vi "AutoFocus Loop.vi"(8 "error in":errorcluster, 9 "IBM OptoElectroMechanics Configuration":T1={"Parameter Analizer"={"Parameter Analyzer VISA Session"="COM1", "Sweeping Time Parameters"={"Integration Time"=0, "Short Integration Time (s)"=1.0, "Long Integration Time (s)"=0.0, "Wait Time Parameter"=1.0}, "Acquisition Mode"=enum."Sweeping Mode", "Status Polling Time (ms)"=0, "Comment"="Test VI", "SMU 1 - Sweeping"={"Start / Offset"=0.0, "Stop / Ratio"=1.0, "Step \n(linear only)"=0.01, "Compliance"=0.1, "Power \nCompliance"=0.0, "Mode"=0, "Function"=0, "Sweep Mode"=FALSE}, "SMU 2 - Sweeping"={"Start / Offset"=0.0, "Stop / Ratio"=1.0, "Step \n(linear only)"=0.01, "Compliance"=0.1, "Power \nCompliance"=0.0, "Mode"=0, "Function"=0, "Sweep Mode"=FALSE}, "SMU 3 - Sweeping"={"Start / Offset"=0.0, "Stop / Ratio"=1.0, "Step \n(linear only)"=0.01, "Compliance"=0.1, "Power \nCompliance"=0.0, "Mode"=0, "Function"=0, "Sweep Mode"=FALSE}, "SMU 4 - Sweeping"={"Start / Offset"=0.0, "Stop / Ratio"=1.0, "Step \n(linear only)"=0.01, "Compliance"=0.1, "Power \nCompliance"=0.0, "Mode"=0, "Function"=0, "Sweep Mode"=FALSE}, "Sweep Spacing"=0, "Range"=0, "SMU1 - Sampling"={"Source"=10.0, "Compliance"=1e-05, "Mode"=0, "Function"=FALSE}, "SMU2 - Sampling"={"Source"=1.0, "Compliance"=1.0, "Mode"=0, "Function"=FALSE}, "SMU3 - Sampling"={"Source"=10.0, "Compliance"=1e-05, "Mode"=0, "Function"=FALSE}, "SMU4 - Sampling"={"Source"=0.1, "Compliance"=60.0, "Mode"=10, "Function"=FALSE}, "Sampling Time Parameters"={"Initial Interval (s)"=0.1, "Number of Samples"=60, "Total Sampling Time (s)"=10.0, "Hold Time (s)"=0.0, "Sampling Mode"=0, "Sampling Time"=0}, "Stop Condition"={"Enable Delay (s)"=0.0, "Name"="", "Threshold"=0.0, "num. of events"=1, "Event"=0, "Stop Condition Enable"=FALSE}}, "Switching Matrix"={"Switching Matrix VISA Session"="GPIB0::18::INSTR", "Connections"=[{"Connections"=[FALSE, FALSE, FALSE, FALSE, FALSE, FALSE, FALSE, FALSE, FALSE, FALSE, FALSE, FALSE], "Connection Type"=enum."Disconnected"}, {"Connections"=[FALSE, FALSE, FALSE, FALSE, FALSE, FALSE, FALSE, FALSE, FALSE, FALSE, FALSE, FALSE], "Connection Type"=enum."Disconnected"}, {"Connections"=[FALSE, FALSE, FALSE, FALSE, FALSE, FALSE, FALSE, FALSE, FALSE, FALSE, FALSE, FALSE], "Connection Type"=enum."Disconnected"}, {"Connections"=[FALSE, FALSE, FALSE, FALSE, FALSE, FALSE, FALSE, FALSE, FALSE, FALSE, FALSE, FALSE], "Connection Type"=enum."Disconnected"}, {"Connections"=[FALSE, FALSE, FALSE, FALSE, FALSE, FALSE, FALSE, FALSE, FALSE, FALSE, FALSE, FALSE], "Connection Type"=enum."Disconnected"}, {"Connections"=[FALSE, FALSE, FALSE, FALSE, FALSE, FALSE, FALSE, FALSE, FALSE, FALSE, FALSE, FALSE], "Connection Type"=enum."Disconnected"}, {"Connections"=[FALSE, FALSE, FALSE, FALSE, FALSE, FALSE, FALSE, FALSE, FALSE, FALSE, FALSE, FALSE], "Connection Type"=enum."Disconnected"}, {"Connections"=[FALSE, FALSE, FALSE, FALSE, FALSE, FALSE, FALSE, FALSE, FALSE, FALSE, FALSE, FALSE], "Connection Type"=enum."Disconnected"}]}, "Stress Control"={"Stress Control VISA Session"="StrainMotor", "Axis"=0, "Motion"=0, "Destination (°)"=0.0, "Speed (°/s)"=4.0, "Position (°)"=25.0}, "Optical Spectrometer"={"Laser Settings"={"Laser Wavelength"=enum."365 nm", "Neutral Density Filter"=enum."100%"}, "Spectrometer Settings"={"Confocal Hole Size (µm)"=0.0, "Grating"=2, "Detector"=enum."InGaAs Array"}, "Acquisition Settings"={"Acquisition Mode"=enum."Multi-Window", "Spectal Position (nm)"=632.0, "From (nm)"=735.0, "To (nm)"=0.0, "Integration Time (s)"=0.0, "Number of Accumulations"=3, "AutoScanning"=FALSE, "Spike Removal"=FALSE}, "Path"=path "C:/07 - Prizes and Awards/Marie Curie Prize/Reply Editors Final NCOMMS(10).docx"}, "Switches & Mirrors"={"Relay VISA Session"="COM1", "Switches"={"Laser"=FALSE, "Video"=FALSE}, "Delays (ms)"={"Laser"=500, "Video"=1500}}, "Camera"={"Settings"={"Pixel clock"=20, "Frame rate"=30.0, "Exposure time"=33.21525, "Master Gain"=0, "Red Gain"=0, "Green Gain"=0, "Blue Gain"=0, "Auto Gain"=FALSE, "White-balance"=FALSE, "Color Correction"=FALSE}}, "XYZ Stage"={"Connection Settings"={"Tango VISA"="", "Baudrate"=57600, "Show Protocol?"=FALSE}, "Manual Control"={"North"=FALSE, "South"=FALSE, "West"=FALSE, "East"=FALSE, "Up"=FALSE, "Down"=FALSE, "Stop"=FALSE, "XY Step"=0.0, "Z step"=0.0}, "Coordinate Control"={"Motion Mode"=enum."Absolute", "Destination [mm]"=[]}}, "AutoFocus"={"Matching Criteria"={"Minimum Score"=700.0, "Color Score Weight"=700.0, "Minimum Contrast"=50, "Match Mode"=0, "Match Feature Mode"=0, "Subpixel Accuracy"=TRUE, "Color Sensitivity"=1, "Search Strategy"=1}, "Z Scan Parameters"={"Z Range"=1380.0, "Resolution"=5000.0, "Initial Direction"=enum."Up", "Focus Threshold"=0.1, "Ascent Constant"=0.1}, "Displacement"=0.0, "Transformation Matrix"=[]}, "Sava Data"={"Workspace Info"={"Device Name"="ProberHead_Tst_C29K3_7(2)", "Device Info"="ProberHead_Tst_C29", "Path"=path "C:/Users/gio/Desktop/ProbeHeadTest"}, "Instrument Configuration"={"Instrument"=enum."Unknown Instrument", "Configuration"="Test Configuration"}, "Stress Motor Position"=0.0, "Electrical Measurement"={"Sequence"=[], "V1"=[], "V2"=[], "V3"=[], "V4"=[], "I1"=[], "I2"=[], "I3"=[], "I4"=[]}, "Optical Spectrum"={"Intensity"=[], "Wavelength"=[], "Energy"=[], "Raman Shift"=[], "Detector Temperature"=0.0}}, "PlotData"={"Sliders"={"Strain Sequence"=0, "Instrument Sequence"=0}, "Measurement"={"Which Instrument?"=enum."No Plot", "Electrical Measurement"={"Sequence"=[], "V1"=[], "V2"=[], "V3"=[], "V4"=[], "I1"=[], "I2"=[], "I3"=[], "I4"=[]}, "Measurement Mode"=enum."Sweeping Mode", "Optical Spectrum"={"Intensity"=[], "Wavelength"=[], "Energy"=[], "Raman Shift"=[], "Detector Temperature"=0.0}}, "Instrument Steps"=[], "Strain Points"=[]}, "Instrument Sequence"={"Caller VI"=enum."User"}, "Strain Measurement"={"Stress Sequence "={"Max Motor Position"=1380.0, "# Intermediate Points"=5000, "Initial Direction"=enum."Tension"}, "Track?"=FALSE}} {"AutoFocus"."Displacement" scale=1.0..1000.0; "AutoFocus"."Z Scan Parameters"."Focus Threshold" min=0.0 max=1000.0 step=1.0 format="%#_2f"; "AutoFocus"."Z Scan Parameters"."Ascent Constant" min=0.0 max=1000.0 step=1.0 format="%#_2f"; "AutoFocus"."Z Scan Parameters"."Resolution" min=0.0 max=1.0 step=0.01 format="%_2g"; "AutoFocus"."Z Scan Parameters"."Z Range" format="%_3g"; "AutoFocus"."Matching Criteria"."Match Mode" items=["Shift Invariant", "Rotation Invariant"]; "AutoFocus"."Matching Criteria"."Match Feature Mode" items=["Color and Shape", "Color", "Shape"]; "AutoFocus"."Matching Criteria"."Color Sensitivity" items=["Low Sensitivity", "Medium Sensitivity", "High Sensitivity"]; "AutoFocus"."Matching Criteria"."Search Strategy" items=["Conservative", "Balance", "Aggressive", "Very Aggressive"]; "XYZ Stage"."Manual Control"."Z step" scale=0.1..10.0; "XYZ Stage"."Manual Control"."XY Step" scale=0.1..1000.0; "Camera"."Settings"."Blue Gain" min=0 max=100 scale=0.0..100.0; "Camera"."Settings"."Green Gain" min=0 max=100 scale=0.0..100.0; "Camera"."Settings"."Red Gain" min=0 max=100 scale=0.0..100.0; "Camera"."Settings"."Master Gain" min=0 max=100 scale=0.0..100.0; "Camera"."Settings"."Exposure time" min=0.101625 max=159.246375 step=0.101625 scale=0.101625..159.246375 scale format="%#.3g"; "Camera"."Settings"."Frame rate" min=2.7455631699174137 max=6.2675785993528725 step=0.000101625 scale=2.7455631699174137..6.2675785993528725 scale format="%^#_3g"; "Camera"."Settings"."Pixel clock" min=5 max=43 scale=5.0..43.0; "PlotData"."Sliders"."Instrument Sequence" scale=0.0..10.0; "PlotData"."Sliders"."Strain Sequence" scale=0.0..10.0; "Strain Measurement"."Stress Sequence"."# Intermediate Points" max=1390; "Parameter Analizer"."Stop Condition"."Event" items=["Value > Threshold", "Value < Threshold", "| Value | > | Threshold |", "| Value | < | Threshold |"]; "Parameter Analizer"."Stop Condition"."Threshold" format="%^.2e"; "Parameter Analizer"."Stop Condition"."Enable Delay (s)" format="%.1f"; "Parameter Analizer"."Sampling Time Parameters"."Sampling Time" items=["Auto (linear only)", "No Limit", "Set Limit"]; "Parameter Analizer"."Sampling Time Parameters"."Sampling Mode" items=["Linear", "Log10", "Log25", "Log50", "Thinned Out"]; "Parameter Analizer"."Sampling Time Parameters"."Hold Time (s)" format="%.4f"; "Parameter Analizer"."Sampling Time Parameters"."Total Sampling Time (s)" format="%.1f"; "Parameter Analizer"."Sampling Time Parameters"."Initial Interval (s)" format="%^.3e"; "Parameter Analizer"."SMU 4 - Sweeping"."Function" items=["Disabled", "Var 1", "Var 2", "Var 1'", "Constant"]; "Parameter Analizer"."SMU 4 - Sweeping"."Mode" items=["V", "I", "V pulse", "I  pulse", "Common"]; "Parameter Analizer"."SMU 4 - Sweeping"."Power \nCompliance" format="%^.2e"; "Parameter Analizer"."SMU 4 - Sweeping"."Compliance" format="%^.2e"; "Parameter Analizer"."SMU 4 - Sweeping"."Step \n(linear only)" format="%^.4e"; "Parameter Analizer"."SMU 4 - Sweeping"."Stop / Ratio" format="%^.4e"; "Parameter Analizer"."SMU 4 - Sweeping"."Start / Offset" format="%^.4e"; "Parameter Analizer"."SMU 3 - Sweeping"."Function" items=["Disabled", "Var 1", "Var 2", "Var 1'", "Constant"]; "Parameter Analizer"."SMU 3 - Sweeping"."Mode" items=["V", "I", "V pulse", "I  pulse", "Common"]; "Parameter Analizer"."SMU 3 - Sweeping"."Power \nCompliance" format="%^.2e"; "Parameter Analizer"."SMU 3 - Sweeping"."Compliance" format="%^.2e"; "Parameter Analizer"."SMU 3 - Sweeping"."Step \n(linear only)" format="%^.4e"; "Parameter Analizer"."SMU 3 - Sweeping"."Stop / Ratio" format="%^.4e"; "Parameter Analizer"."SMU 3 - Sweeping"."Start / Offset" format="%^.4e"; "Parameter Analizer"."SMU 2 - Sweeping"."Function" items=["Disabled", "Var 1", "Var 2", "Var 1'", "Constant"]; "Parameter Analizer"."SMU 2 - Sweeping"."Mode" items=["V", "I", "V pulse", "I  pulse", "Common"]; "Parameter Analizer"."SMU 2 - Sweeping"."Power \nCompliance" format="%^.2e"; "Parameter Analizer"."SMU 2 - Sweeping"."Compliance" format="%^.2e"; "Parameter Analizer"."SMU 2 - Sweeping"."Step \n(linear only)" format="%^.4e"; "Parameter Analizer"."SMU 2 - Sweeping"."Stop / Ratio" format="%^.4e"; "Parameter Analizer"."SMU 2 - Sweeping"."Start / Offset" format="%^.4e"; "Parameter Analizer"."SMU 1 - Sweeping"."Function" items=["Disabled", "Var 1", "Var 2", "Var 1'", "Constant"]; "Parameter Analizer"."SMU 1 - Sweeping"."Mode" items=["V", "I", "V pulse", "I  pulse", "Common"]; "Parameter Analizer"."SMU 1 - Sweeping"."Power \nCompliance" format="%^.2e"; "Parameter Analizer"."SMU 1 - Sweeping"."Compliance" format="%^.2e"; "Parameter Analizer"."SMU 1 - Sweeping"."Step \n(linear only)" format="%^.4e"; "Parameter Analizer"."SMU 1 - Sweeping"."Stop / Ratio" format="%^.4e"; "Parameter Analizer"."SMU 1 - Sweeping"."Start / Offset" format="%^.4e"; "Parameter Analizer"."Sweeping Time Parameters"."Long Integration Time (s)" scale=0.02..2.0; "Parameter Analizer"."Sweeping Time Parameters"."Short Integration Time (s)" scale=8e-05..0.00192; "Parameter Analizer"."Sweeping Time Parameters"."Integration Time" items=["Short", "Long"]; "Parameter Analizer"."Sweeping Time Parameters"."Wait Time Parameter" format="%.1f"; "Parameter Analizer"."SMU4 - Sampling"."Mode" items=["V", "I", "Common"]; "Parameter Analizer"."SMU4 - Sampling"."Compliance" format="%^.2e"; "Parameter Analizer"."SMU4 - Sampling"."Source" format="%^.3e"; "Parameter Analizer"."SMU3 - Sampling"."Mode" items=["V", "I", "Common"]; "Parameter Analizer"."SMU3 - Sampling"."Compliance" format="%^.2e"; "Parameter Analizer"."SMU3 - Sampling"."Source" format="%^.3e"; "Parameter Analizer"."SMU2 - Sampling"."Mode" items=["V", "I", "Common"]; "Parameter Analizer"."SMU2 - Sampling"."Compliance" format="%^.2e"; "Parameter Analizer"."SMU2 - Sampling"."Source" format="%^.3e"; "Parameter Analizer"."SMU1 - Sampling"."Mode" items=["V", "I", "Common"]; "Parameter Analizer"."SMU1 - Sampling"."Compliance" format="%^.2e"; "Parameter Analizer"."SMU1 - Sampling"."Source" format="%^.3e"; "Parameter Analizer"."Range" items=["auto", "fixed", "limited"]; "Parameter Analizer"."Sweep Spacing" items=["linear", "log 10", "log 25", "log 50"]; "Stress Control"."Axis" min=1 max=3; "Stress Control"."Position (°)" format="%.6g"; "Stress Control"."Speed (°/s)" min=0.0 max=4.0 format="%.6f"; "Stress Control"."Destination (°)" min=-2000000000.0 max=2000000000.0 format="%.6f"; "Stress Control"."Motion" items=["Absolute", "Relative"]; "Optical Spectrometer"."Spectrometer Settings"."Grating" items=["1800 l/mm", "150 l/mm"]}, 10 "Message Queues out":T57, 11 "Notifiers":T44) -> (0 "error out":errorcluster)   [LabVIEW 2014]
uses:
  support/Message Queue/All Message Queues.ctl
  support/Message Queue/Message Cluster.ctl
  support/Notifiers/Notifiers.ctl
  support/Message Handler Loop Notifiers.ctl
  Hardware Control/Parameter Analyzer/Parameter Analyzer Notifiers.ctl
  Hardware Control/Switching Matrix/Switching Matrix Notifiers.ctl
  Hardware Control/Stress Control/StressControl Notifiers.ctl
  Hardware Control/Spectrometer/Spectrometer Notifiers.ctl
  Hardware Control/Switches and Mirrors/SwitchesMirrors Notifiers.ctl
  Hardware Control/Camera/Camera Notifiers.ctl
  Hardware Control/XYZ Stage/XYZ Notifications.ctl
  Hardware Control/Autofocus/Autofocus Notifiers.ctl
  Measurements/Optoelectronic Measurement/Optoelectronic Notifiers.ctl
  Measurements/Save Data/SaveData Notifiers.ctl
  Measurements/Instrument Sequence/Instrument Sequence Notifiers.ctl
  support/Configuration/Configuration.ctl
  Hardware Control/Parameter Analyzer/Parameter Analyzer Config.ctl
  Hardware Control/Parameter Analyzer/Parameter Analyzer Integration Parameters.ctl
  Hardware Control/Parameter Analyzer/Parameter Analyzer SMU Sweeping.ctl
  Hardware Control/Parameter Analyzer/Parameter Analyzer Sweep Spacing.ctl
  Hardware Control/Parameter Analyzer/Parameter Analyzer SMU Range.ctl
  Hardware Control/Parameter Analyzer/Parameter Analyzer SMU Sampling.ctl
  Hardware Control/Parameter Analyzer/Parameter Analyzer Sampling Parameters.ctl
  Hardware Control/Parameter Analyzer/Parameter Analyzer Stop Sampling Conditions.ctl
  Hardware Control/Switching Matrix/Switching Matrix Config.ctl
  Hardware Control/Stress Control/StressControl Config.ctl
  Hardware Control/Spectrometer/Spectrometer Config.ctl
  Hardware Control/Spectrometer/Laser Settings.ctl
  Hardware Control/Spectrometer/Laser.ctl
  Hardware Control/Spectrometer/Filter.ctl
  Hardware Control/Spectrometer/Grating Detector Settings.ctl
  Hardware Control/Spectrometer/Grating.ctl
  Hardware Control/Spectrometer/Detector.ctl
  Hardware Control/Spectrometer/Acquisition Settings.ctl
  Hardware Control/Switches and Mirrors/SwitchesMirrors Config.ctl
  Hardware Control/Switches and Mirrors/SwitchesMirrors Status.ctl
  Hardware Control/Camera/Camera Config.ctl
  Hardware Control/Camera/Camera Settings.ctl
  Hardware Control/XYZ Stage/XYZ Config.ctl
  Hardware Control/XYZ Stage/XYZ Connection Settings.ctl
  Hardware Control/XYZ Stage/XYZ Stage Control.ctl
  Hardware Control/XYZ Stage/XYZ Coordinate Control.ctl
  Hardware Control/Autofocus/AutoFocus Config.ctl
  Hardware Control/Autofocus/ZScan.ctl
  <vilib>/Analysis/Matrix/Datatypes/RealMatrix.ctl
  Measurements/Save Data/SaveData Config.ctl
  Measurements/Save Data/SaveData Workspace Info.ctl
  Measurements/Save Data/SaveData Instrument Configuration.ctl
  Measurements/Instrument Sequence/Instrument List.ctl
  Hardware Control/Spectrometer/Spectral Data.ctl
  Measurements/Plot Data/PlotData Config.ctl
  Measurements/Plot Data/Measurement.ctl
  Measurements/Plot Data/WhichInstrument.ctl
  Hardware Control/Parameter Analyzer/Electrical Data.ctl
  Measurements/Instrument Sequence/Instrument Steps.ctl
  Measurements/Instrument Sequence/Action.ctl
  Measurements/Instrument Sequence/Instrument Sequence Config.ctl
  Measurements/Strain Measurement/Strain Measurement Config.ctl
  Hardware Control/Autofocus/AutoFocus Functions.ctl
  support/Message Queue/Message Queue.lvlib
  <vilib>/Analysis/Matrix/NI_Matrix.lvlib
panel:
  # "LICENSED MATERIALS – PROPERTY OF IBM\nCopyright IBM Corp. 2016,\nALL RIGHTS RESERVED"
  # "XY"
  # "Z"
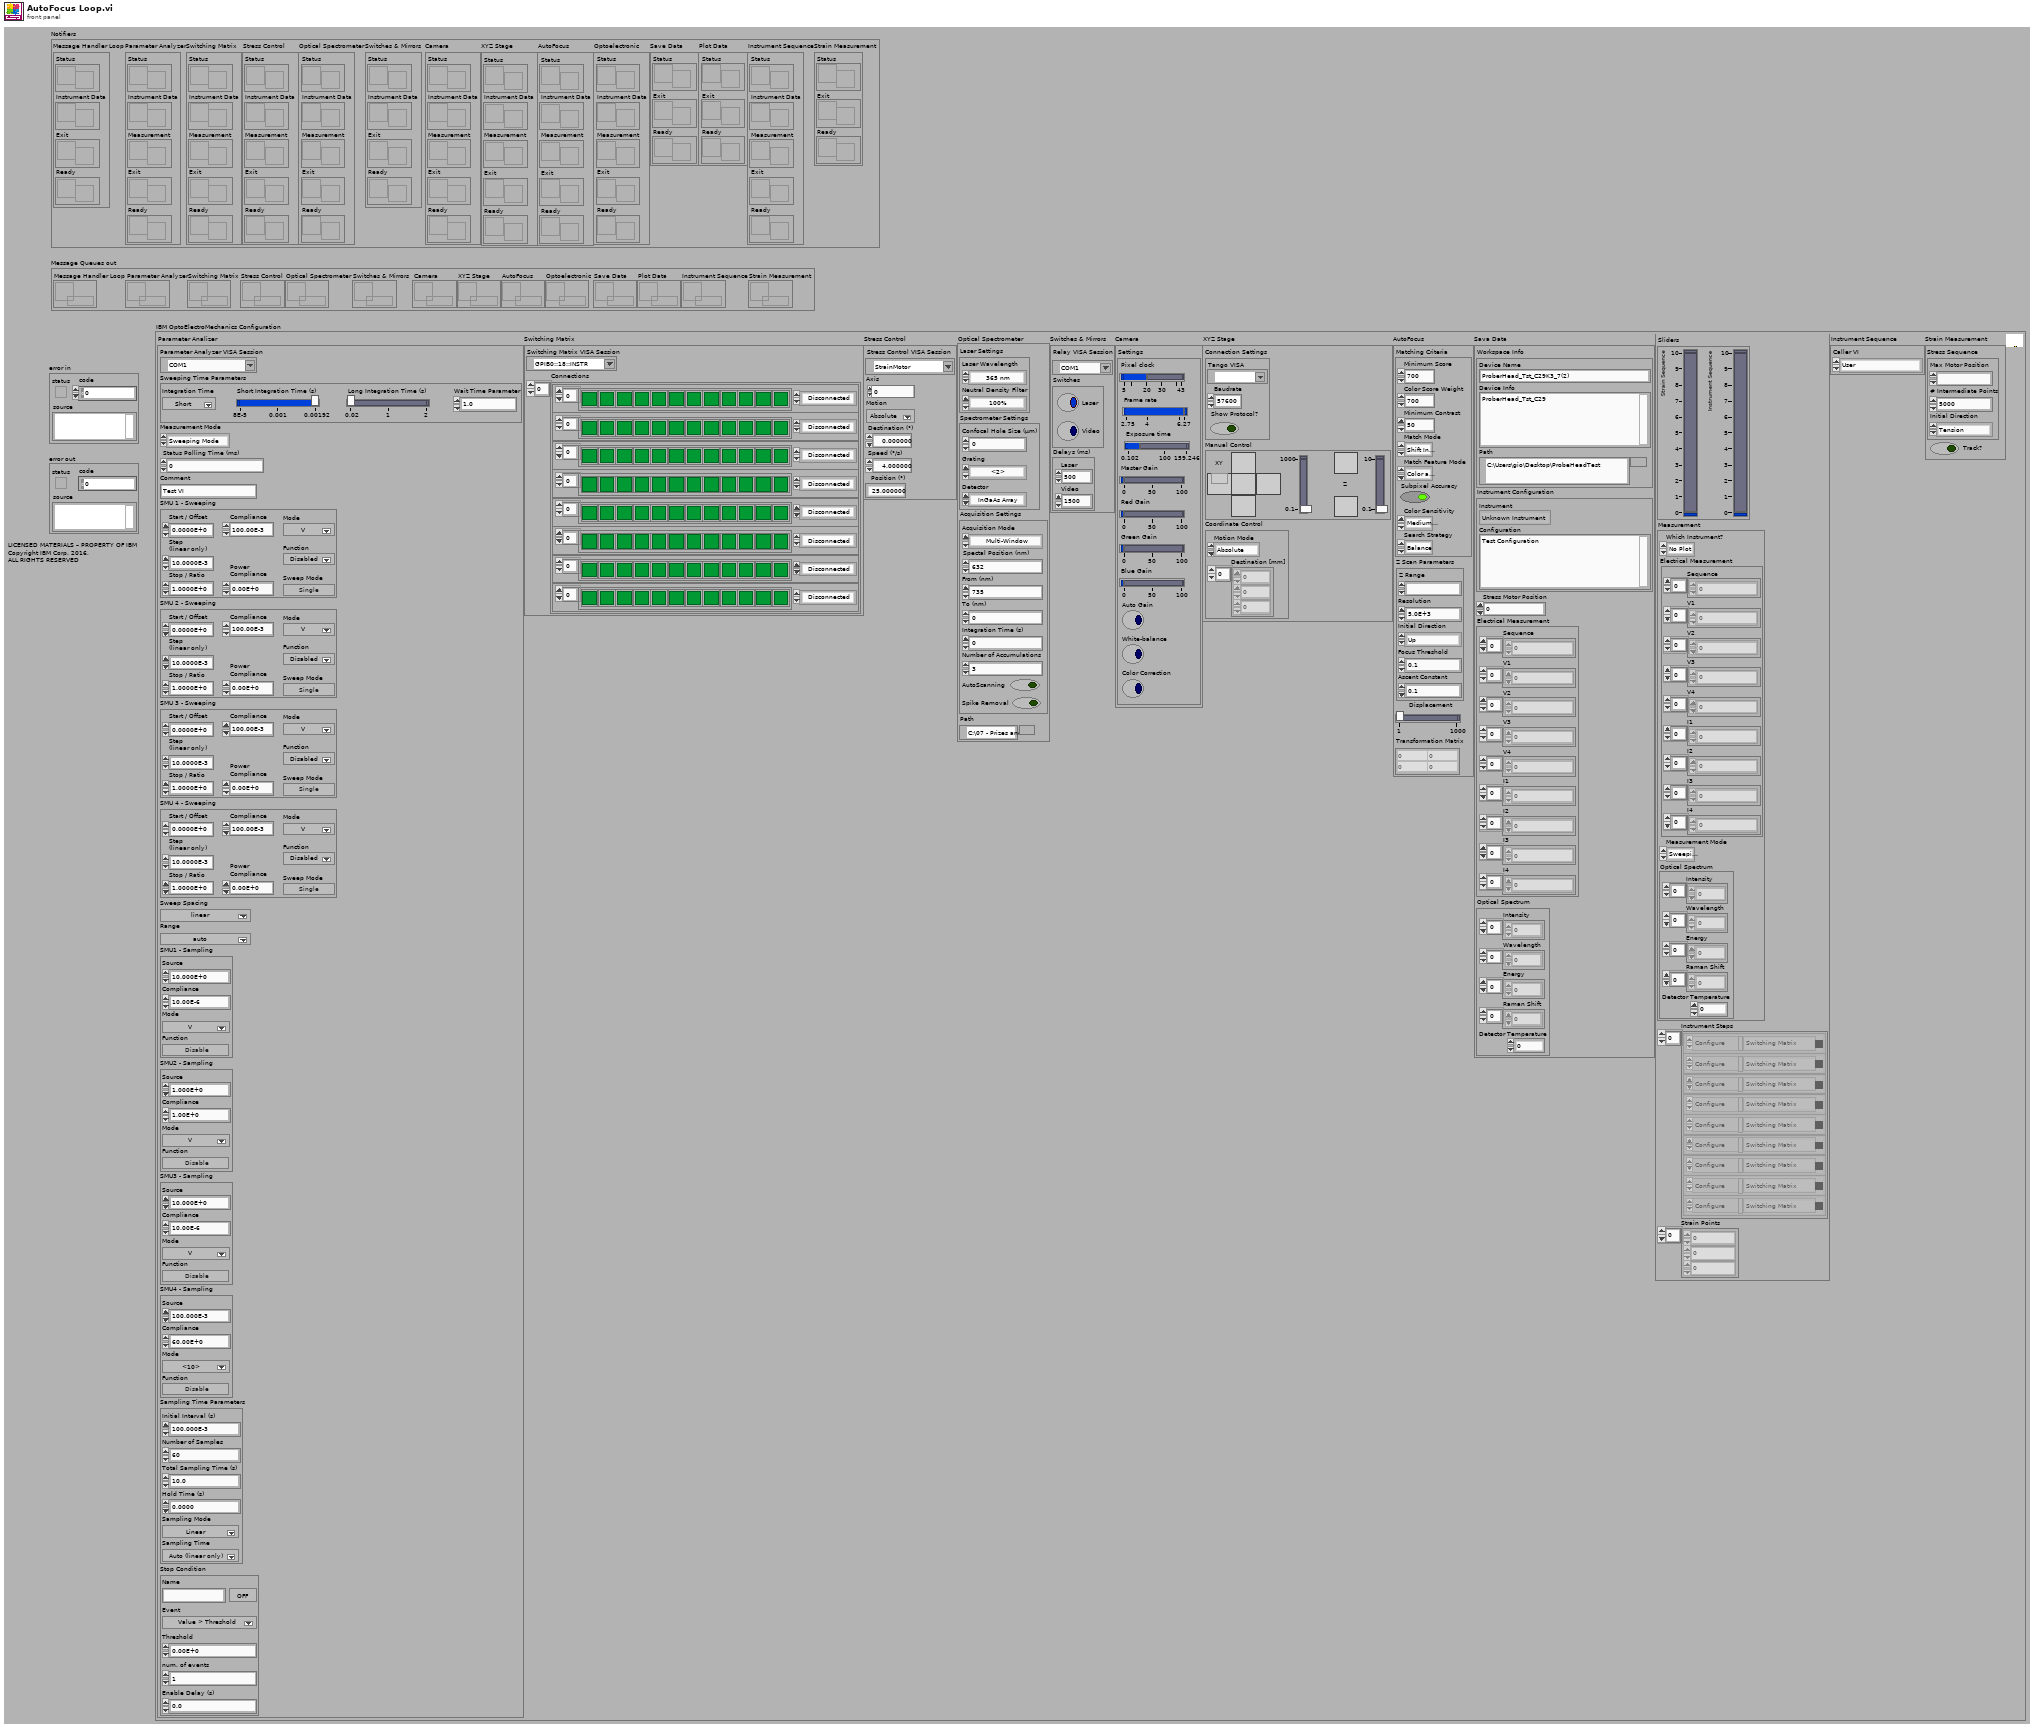
[diagram p1: front panel]
types:
  T1 = typedef "Configuration.ctl" = cluster{"Parameter Analizer":T2, "Switching Matrix":T10, "Stress Control":T11, "Optical Spectrometer":T12, "Switches & Mirrors":T20, "Camera":T22, "XYZ Stage":T24, "AutoFocus":T28, "Sava Data":T31, "PlotData":T36, "Instrument Sequence":T42, "Strain Measurement":T43}
  T2 = typedef "Parameter Analyzer Config.ctl" = cluster{"Parameter Analyzer VISA Session":refnum<visa-resource-name>, "Sweeping Time Parameters":T3, "Acquisition Mode":enum32{"Sweeping Mode", "Sampling Mode"}, "Status Polling Time (ms)":u32, "Comment":string, "SMU 1 - Sweeping":T4, "SMU 2 - Sweeping":T4, "SMU 3 - Sweeping":T4, "SMU 4 - Sweeping":T4, "Sweep Spacing":T5, "Range":T6, "SMU1 - Sampling":T7, "SMU2 - Sampling":T7, "SMU3 - Sampling":T7, "SMU4 - Sampling":T7, "Sampling Time Parameters":T8, "Stop Condition":T9}
  T3 = typedef "Parameter Analyzer Integration Parameters.ctl" = cluster{"Integration Time":u32, "Short Integration Time (s)":dbl, "Long Integration Time (s)":dbl, "Wait Time Parameter":dbl}
  T4 = typedef "Parameter Analyzer SMU Sweeping.ctl" = cluster{"Start / Offset":dbl, "Stop / Ratio":dbl, "Step \n(linear only)":dbl, "Compliance":dbl, "Power \nCompliance":dbl, "Mode":u32, "Function":i32, "Sweep Mode":bool}
  T5 = typedef "Parameter Analyzer Sweep Spacing.ctl" = u16
  T6 = typedef "Parameter Analyzer SMU Range.ctl" = u16
  T7 = typedef "Parameter Analyzer SMU Sampling.ctl" = cluster{"Source":dbl, "Compliance":dbl, "Mode":u32, "Function":bool}
  T8 = typedef "Parameter Analyzer Sampling Parameters.ctl" = cluster{"Initial Interval (s)":dbl, "Number of Samples":i32, "Total Sampling Time (s)":dbl, "Hold Time (s)":dbl, "Sampling Mode":i32, "Sampling Time":i32}
  T9 = typedef "Parameter Analyzer Stop Sampling Conditions.ctl" = cluster{"Enable Delay (s)":dbl, "Name":string, "Threshold":dbl, "num. of events":i32, "Event":i32, "Stop Condition Enable":bool}
  T10 = typedef "Switching Matrix Config.ctl" = cluster{"Switching Matrix VISA Session":refnum<visa-resource-name>, "Connections":cluster{"Connections":bool[], "Connection Type":enum16{"Disconnected", "Make - Break", "Break - Make"}}[]}
  T11 = typedef "StressControl Config.ctl" = cluster{"Stress Control VISA Session":refnum<visa-resource-name>, "Axis":i32, "Motion":u16, "Destination (°)":dbl, "Speed (°/s)":dbl, "Position (°)":dbl}
  T12 = typedef "Spectrometer Config.ctl" = cluster{"Laser Settings":T13, "Spectrometer Settings":T16, "Acquisition Settings":T19, "Path":path}
  T13 = typedef "Laser Settings.ctl" = cluster{"Laser Wavelength":T14, "Neutral Density Filter":T15}
  T14 = typedef "Laser.ctl" = enum16{"633 nm", "784 nm", "532 nm", "365 nm"}
  T15 = typedef "Filter.ctl" = enum16{"100%", "50%", "25%", "10%", "1%", "0.1%", "0.01%"}
  T16 = typedef "Grating Detector Settings.ctl" = cluster{"Confocal Hole Size (µm)":dbl, "Grating":T17, "Detector":T18}
  T17 = typedef "Grating.ctl" = u16
  T18 = typedef "Detector.ctl" = enum16{"InGaAs Array", "Silicon CCD"}
  T19 = typedef "Acquisition Settings.ctl" = cluster{"Acquisition Mode":enum16{"Single Window", "Multi-Window"}, "Spectal Position (nm)":dbl, "From (nm)":dbl, "To (nm)":dbl, "Integration Time (s)":dbl, "Number of Accumulations":i32, "AutoScanning":bool, "Spike Removal":bool}
  T20 = typedef "SwitchesMirrors Config.ctl" = cluster{"Relay VISA Session":refnum<visa-resource-name>, "Switches":T21, "Delays (ms)":cluster{"Laser":u32, "Video":u32}}
  T21 = typedef "SwitchesMirrors Status.ctl" = cluster{"Laser":bool, "Video":bool}
  T22 = typedef "Camera Config.ctl" = cluster{"Settings":T23}
  T23 = typedef "Camera Settings.ctl" = cluster{"Pixel clock":i32, "Frame rate":dbl, "Exposure time":dbl, "Master Gain":i32, "Red Gain":i32, "Green Gain":i32, "Blue Gain":i32, "Auto Gain":bool, "White-balance":bool, "Color Correction":bool}
  T24 = typedef "XYZ Config.ctl" = cluster{"Connection Settings":T25, "Manual Control":T26, "Coordinate Control":T27}
  T25 = typedef "XYZ Connection Settings.ctl" = cluster{"Tango VISA":refnum<visa-resource-name>, "Baudrate":i32, "Show Protocol?":bool}
  T26 = typedef "XYZ Stage Control.ctl" = cluster{"North":bool, "South":bool, "West":bool, "East":bool, "Up":bool, "Down":bool, "Stop":bool, "XY Step":dbl, "Z step":dbl}
  T27 = typedef "XYZ Coordinate Control.ctl" = cluster{"Motion Mode":enum16{"Absolute", "Relative"}, "Destination [mm]":dbl[]}
  T28 = typedef "AutoFocus Config.ctl" = cluster{"Matching Criteria":cluster{"Minimum Score":sgl, "Color Score Weight":sgl, "Minimum Contrast":i32, "Match Mode":u32, "Match Feature Mode":u32, "Subpixel Accuracy":bool, "Color Sensitivity":u32, "Search Strategy":u32}, "Z Scan Parameters":T29, "Displacement":dbl, "Transformation Matrix":T30}
  T29 = typedef "ZScan.ctl" = cluster{"Z Range":ext, "Resolution":dbl, "Initial Direction":enum16{"Up", "Down"}, "Focus Threshold":dbl, "Ascent Constant":dbl}
  T30 = typedef "NI_Matrix.lvlib/RealMatrix.ctl" = dbl[][]
  T31 = typedef "SaveData Config.ctl" = cluster{"Workspace Info":T32, "Instrument Configuration":T33, "Stress Motor Position":dbl, "Electrical Measurement":cluster{"Sequence":dbl[], "V1":dbl[], "V2":dbl[], "V3":dbl[], "V4":dbl[], "I1":dbl[], "I2":dbl[], "I3":dbl[], "I4":dbl[]}, "Optical Spectrum":T35}
  T32 = typedef "SaveData Workspace Info.ctl" = cluster{"Device Name":string, "Device Info":string, "Path":path}
  T33 = typedef "SaveData Instrument Configuration.ctl" = cluster{"Instrument":T34, "Configuration":string}
  T34 = typedef "Instrument List.ctl" = enum32{"Unknown Instrument", "Switching Matrix", "Parameter Analyzer", "Optical Spectrometer", "Optoelectronic", "Autofocus"}
  T35 = typedef "Spectral Data.ctl" = cluster{"Intensity":dbl[], "Wavelength":dbl[], "Energy":dbl[], "Raman Shift":dbl[], "Detector Temperature":dbl}
  T36 = typedef "PlotData Config.ctl" = cluster{"Sliders":cluster{"Strain Sequence":i32, "Instrument Sequence":i32}, "Measurement":T37, "Instrument Steps":T40, "Strain Points":dbl[]}
  T37 = typedef "Measurement.ctl" = cluster{"Which Instrument?":T38, "Electrical Measurement":T39, "Measurement Mode":enum16{"Sweeping Mode", "Sampling Mode"}, "Optical Spectrum":T35}
  T38 = typedef "WhichInstrument.ctl" = enum16{"No Plot", "Spectrometer", "Parameter Analyzer", "Optoelectronic"}
  T39 = typedef "Electrical Data.ctl" = cluster{"Sequence":dbl[], "V1":dbl[], "V2":dbl[], "V3":dbl[], "V4":dbl[], "I1":dbl[], "I2":dbl[], "I3":dbl[], "I4":dbl[]}
  T40 = typedef "Instrument Steps.ctl" = cluster{"Action":T41, "Configuration":variant, "Instrument":T34, "Status":enum8{"False", "True", "Mixed"}}[]
  T41 = typedef "Action.ctl" = enum32{"Configure", "Measure"}
  T42 = typedef "Instrument Sequence Config.ctl" = cluster{"Caller VI":enum16{"User", "Stress Measurement VI"}}
  T43 = typedef "Strain Measurement Config.ctl" = cluster{"Stress Sequence ":cluster{"Max Motor Position":ext, "# Intermediate Points":u32, "Initial Direction":enum16{"Tension", "Compression"}}, "Track?":bool}
  T44 = typedef "Notifiers.ctl" = cluster{"Message Handler Loop":T45, "Parameter Analyzer":T46, "Switching Matrix":T47, "Stress Control":T48, "Optical Spectrometer":T49, "Switches & Mirrors":T50, "Camera":T51, "XYZ Stage":T52, "AutoFocus":T53, "Optoelectronic":T54, "Save Data":T55, "Plot Data":T55, "Instrument Sequence":T56, "Strain Measurement":cluster{"Status":refnum<notifier>, "Exit":refnum<notifier>, "Ready":refnum<notifier>}}
  T45 = typedef "Message Handler Loop Notifiers.ctl" = cluster{"Status":refnum<notifier>, "Instrument Data":refnum<notifier>, "Exit":refnum<notifier>, "Ready":refnum<notifier>}
  T46 = typedef "Parameter Analyzer Notifiers.ctl" = cluster{"Status":refnum<notifier>, "Instrument Data":refnum<notifier>, "Measurement":refnum<notifier>, "Exit":refnum<notifier>, "Ready":refnum<notifier>}
  T47 = typedef "Switching Matrix Notifiers.ctl" = cluster{"Status":refnum<notifier>, "Instrument Data":refnum<notifier>, "Measurement":refnum<notifier>, "Exit":refnum<notifier>, "Ready":refnum<notifier>}
  T48 = typedef "StressControl Notifiers.ctl" = cluster{"Status":refnum<notifier>, "Instrument Data":refnum<notifier>, "Measurement":refnum<notifier>, "Exit":refnum<notifier>, "Ready":refnum<notifier>}
  T49 = typedef "Spectrometer Notifiers.ctl" = cluster{"Status":refnum<notifier>, "Instrument Data":refnum<notifier>, "Measurement":refnum<notifier>, "Exit":refnum<notifier>, "Ready":refnum<notifier>}
  T50 = typedef "SwitchesMirrors Notifiers.ctl" = cluster{"Status":refnum<notifier>, "Instrument Data":refnum<notifier>, "Exit":refnum<notifier>, "Ready":refnum<notifier>}
  T51 = typedef "Camera Notifiers.ctl" = cluster{"Status":refnum<notifier>, "Instrument Data":refnum<notifier>, "Measurement":refnum<notifier>, "Exit":refnum<notifier>, "Ready":refnum<notifier>}
  T52 = typedef "XYZ Notifications.ctl" = cluster{"Status":refnum<notifier>, "Instrument Data":refnum<notifier>, "Measurement":refnum<notifier>, "Exit":refnum<notifier>, "Ready":refnum<notifier>}
  T53 = typedef "Autofocus Notifiers.ctl" = cluster{"Status":refnum<notifier>, "Instrument Data":refnum<notifier>, "Measurement":refnum<notifier>, "Exit":refnum<notifier>, "Ready":refnum<notifier>}
  T54 = typedef "Optoelectronic Notifiers.ctl" = cluster{"Status":refnum<notifier>, "Instrument Data":refnum<notifier>, "Measurement":refnum<notifier>, "Exit":refnum<notifier>, "Ready":refnum<notifier>}
  T55 = typedef "SaveData Notifiers.ctl" = cluster{"Status":refnum<notifier>, "Exit":refnum<notifier>, "Ready":refnum<notifier>}
  T56 = typedef "Instrument Sequence Notifiers.ctl" = cluster{"Status":refnum<notifier>, "Instrument Data":refnum<notifier>, "Measurement":refnum<notifier>, "Exit":refnum<notifier>, "Ready":refnum<notifier>}
  T57 = typedef "Message Queue.lvlib/All Message Queues.ctl" = cluster{"Message Handler Loop":refnum<queue>, "Parameter Analyzer":refnum<queue>, "Switching Matrix":refnum<queue>, "Stress Control":refnum<queue>, "Optical Spectrometer":refnum<queue>, "Switches & Mirrors":refnum<queue>, "Camera":refnum<queue>, "XYZ Stage":refnum<queue>, "AutoFocus":refnum<queue>, "Optoelectronic":refnum<queue>, "Save Data":refnum<queue>, "Plot Data":refnum<queue>, "Instrument Sequence":refnum<queue>, "Strain Measurement":refnum<queue>}
  T58 = typedef "AutoFocus Data.ctl" = cluster{"Configuration":T28, "Refnums":T59, "Initialize":T61}
  T59 = typedef "AutoFocus Refnums.ctl" = cluster{"Instrument Status":refnum<vi>, "Matching Criteria":refnum<vi>, "Z Scan Parameters":refnum<vi>, "Distance":refnum<vi>, "Transformation Matrix":refnum<vi>, "Match and Edge":T60, "Matching Curves":refnum<vi>, "Tracking":refnum<vi>, "Focus":refnum<vi>, "Find Focus":refnum<vi>, "Set Target":refnum<vi>, "Link Stage & Camera":refnum<vi>, "Align":refnum<vi>}
  T60 = typedef "Target Refnums.ctl" = cluster{"Image":refnum<vi>, "Target":refnum<vi>, "Edge":refnum<vi>, "Target Data":refnum<vi>}
  T61 = typedef "AutoFocus Initialize.ctl" = cluster{"Update Refnums":bool, "Allocate Image Memory":bool, "Set Match Criteria":bool, "Link Stage & Camera":bool, "Set Target":bool, "Find Target":bool}
  T62 = typedef "AutoFocus Functions.ctl" = enum16{"Allocate Image Memory", "Free Image Memory", "Grab Image", "Get ROI", "Set ROI", "Set Match Criteria", "Set Target", "Link Stage & Camera", "Set Transformation Matrix", "Find Target", "Align", "Find Focus", "Focus (Gradient)", "Focus (Threshold)", "Focus (Turning Points)", "Update Refnums"}
  T63 = cluster{"Minimum Score":sgl, "Color Score Weight":sgl, "Minimum Contrast":i32, "Match Mode":u32, "Match Feature Mode":u32, "Subpixel Accuracy":bool, "Color Sensitivity":u32, "Search Strategy":u32}
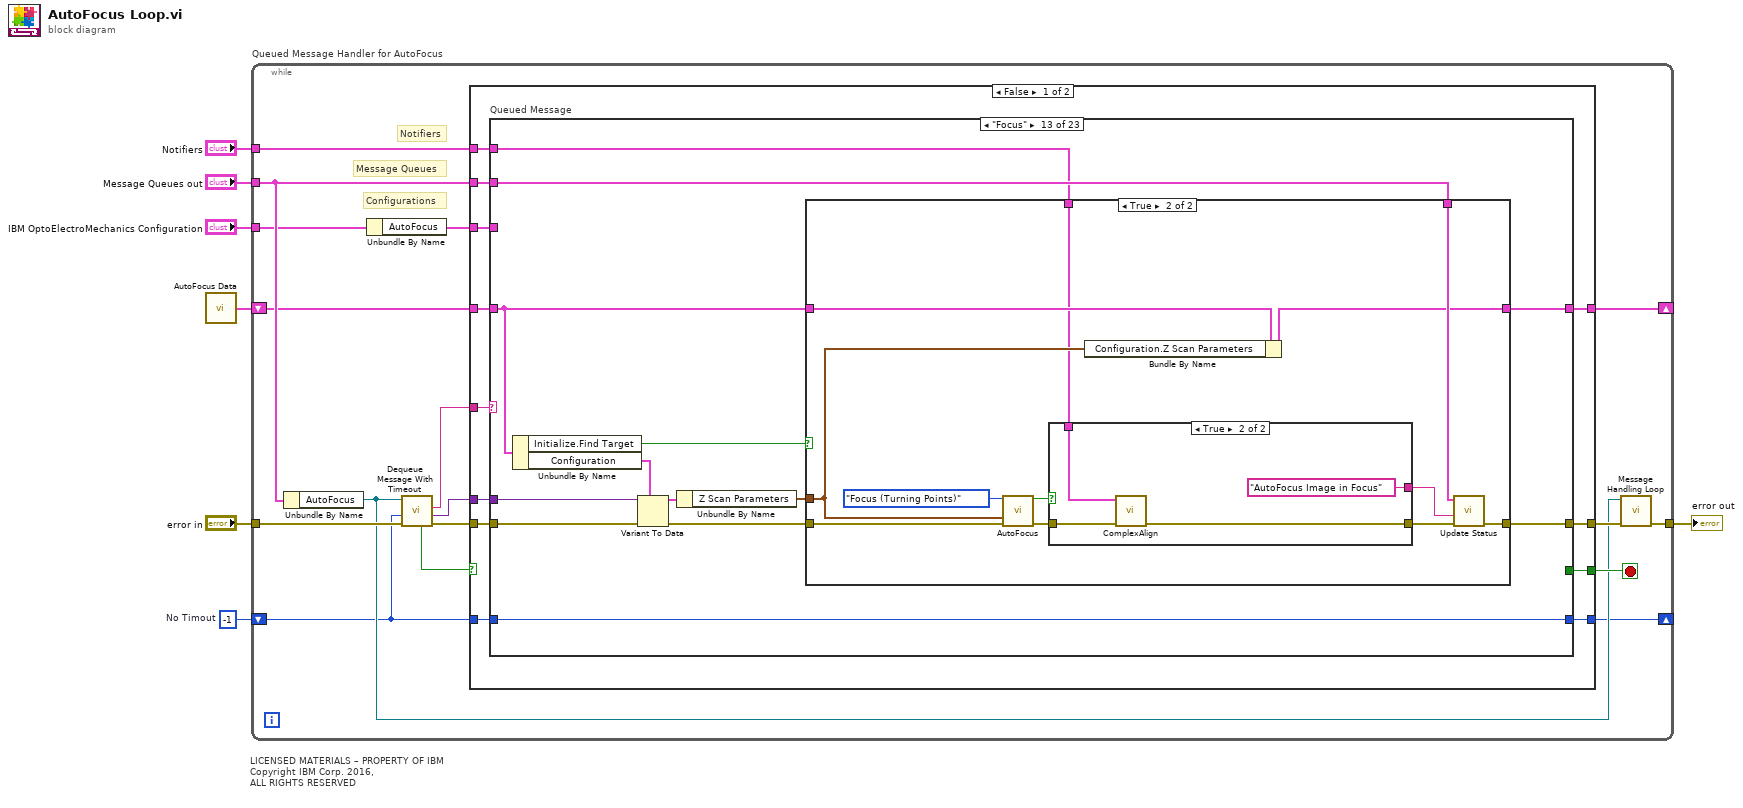
[diagram p0: block diagram]
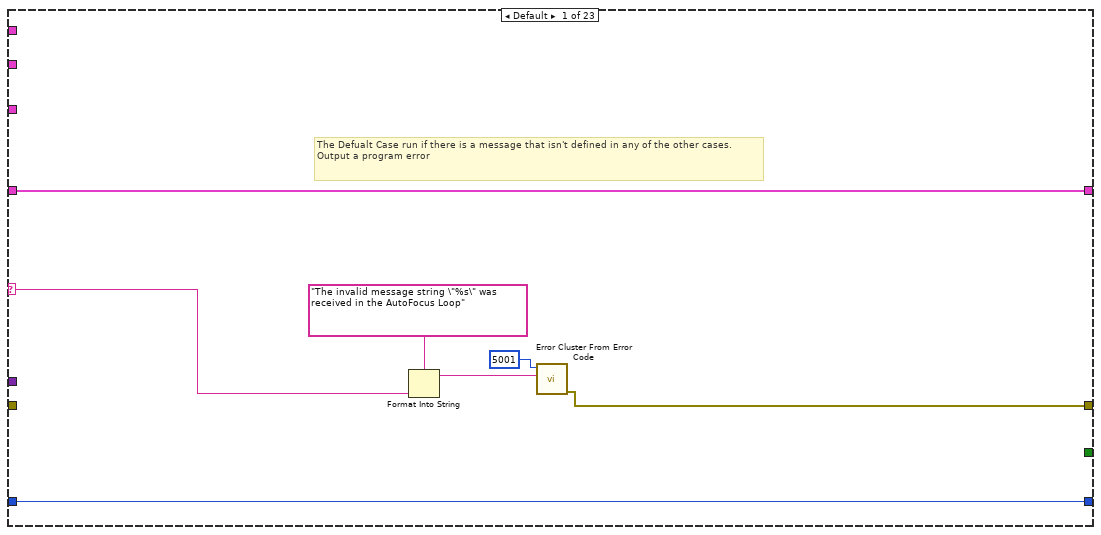
[diagram p2: hidden frame]
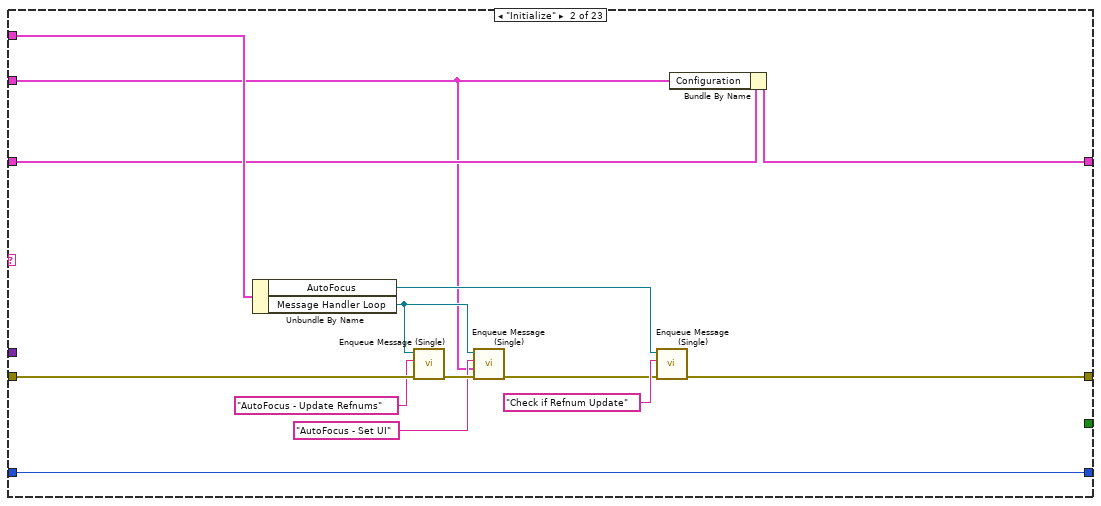
[diagram p3: hidden frame]
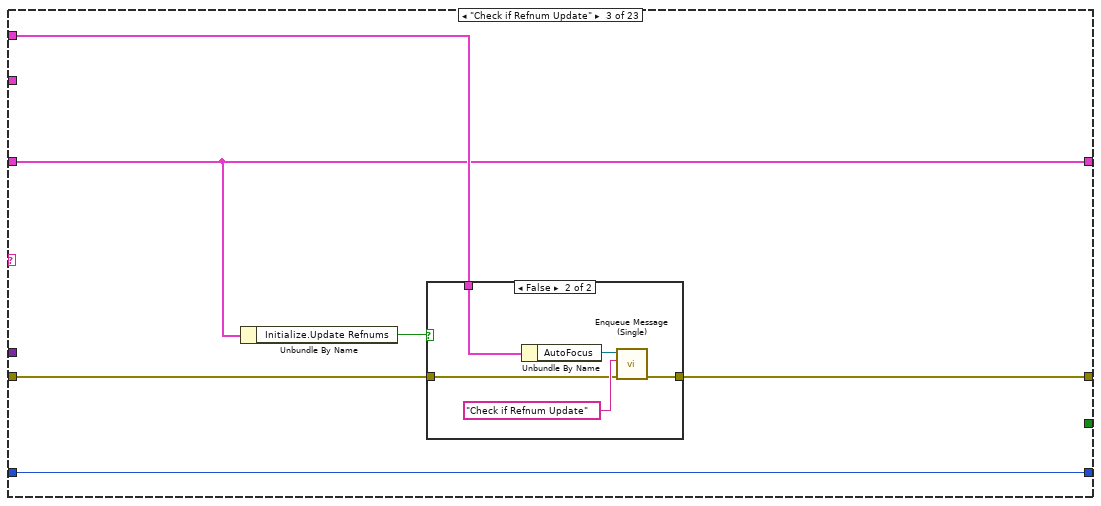
[diagram p4: hidden frame]
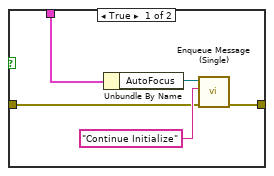
[diagram p5: hidden frame]
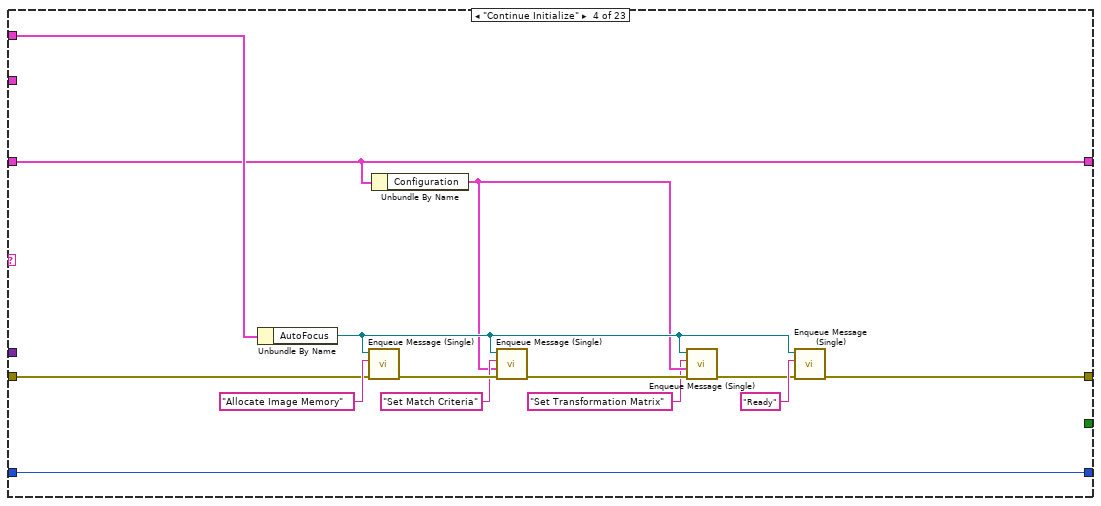
[diagram p6: hidden frame]
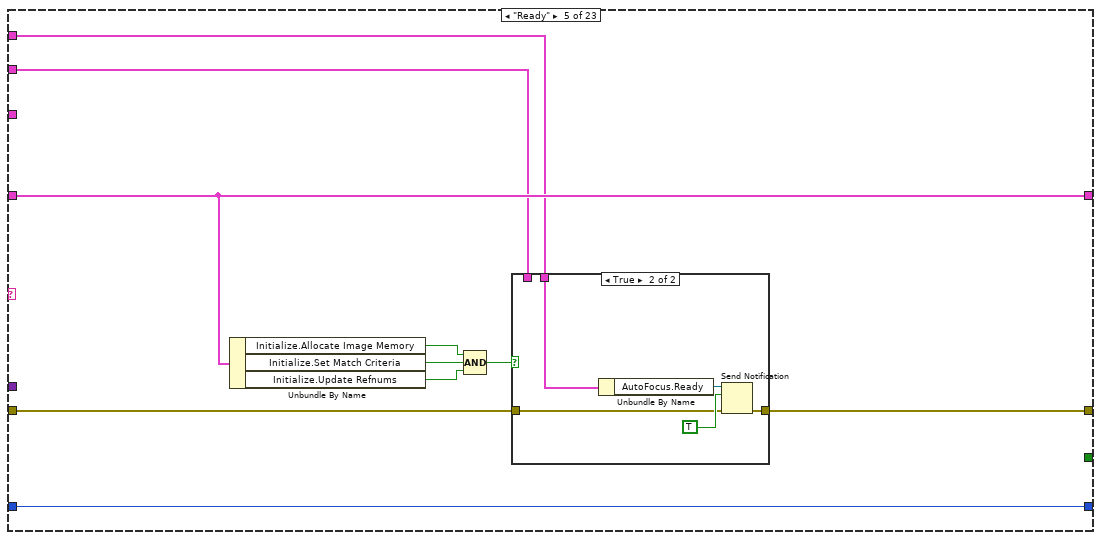
[diagram p7: hidden frame]
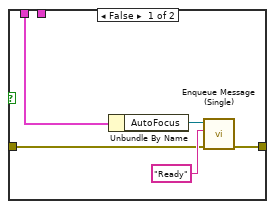
[diagram p8: hidden frame]
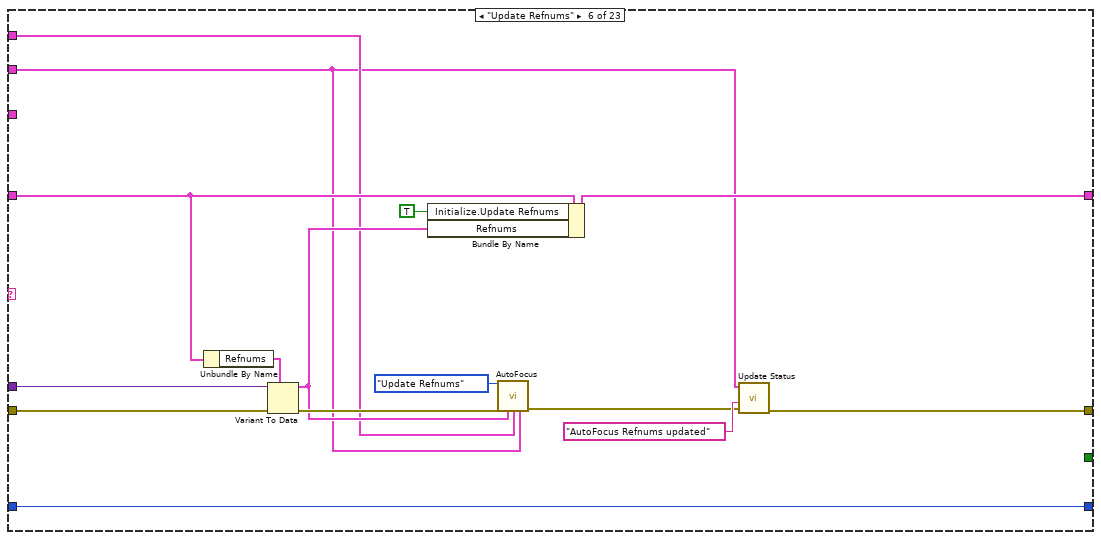
[diagram p9: hidden frame]
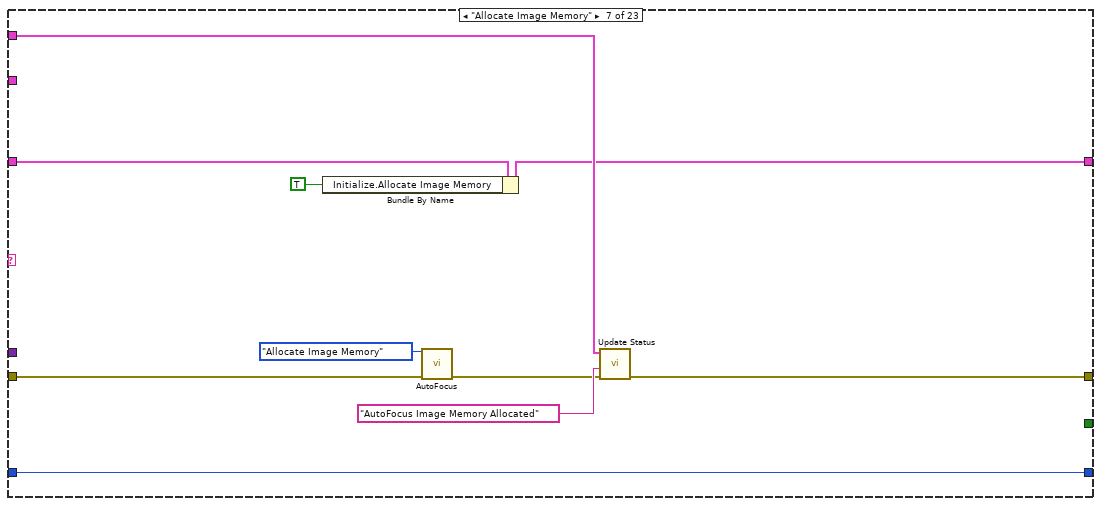
[diagram p10: hidden frame]
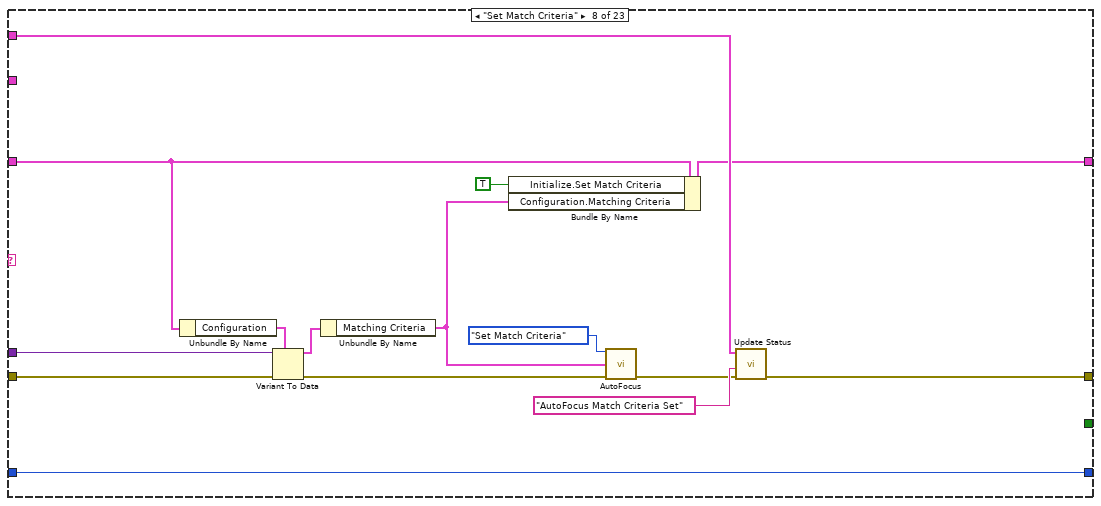
[diagram p11: hidden frame]
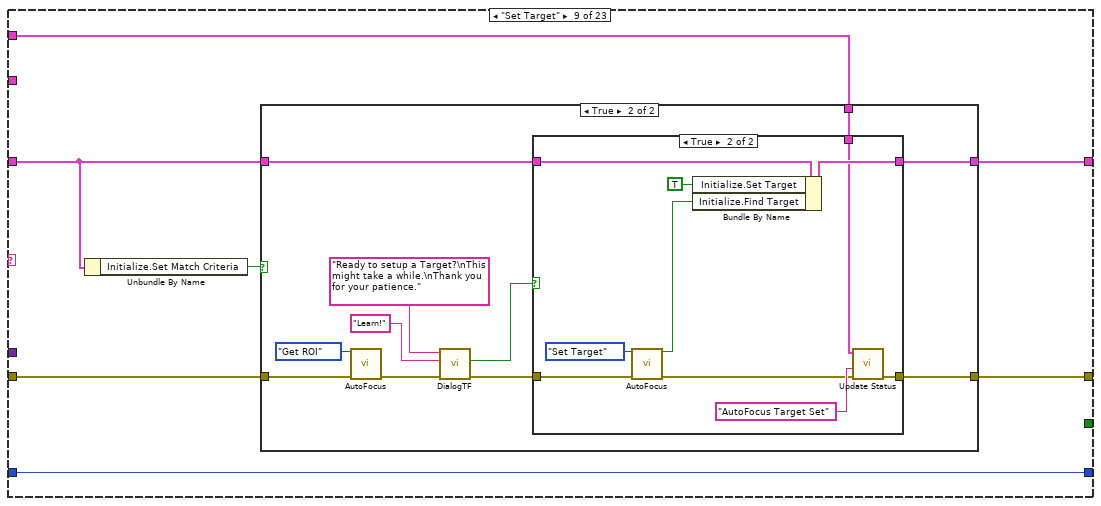
[diagram p12: hidden frame]
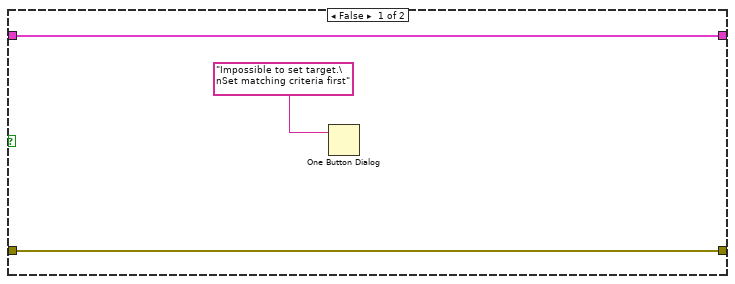
[diagram p13: hidden frame]
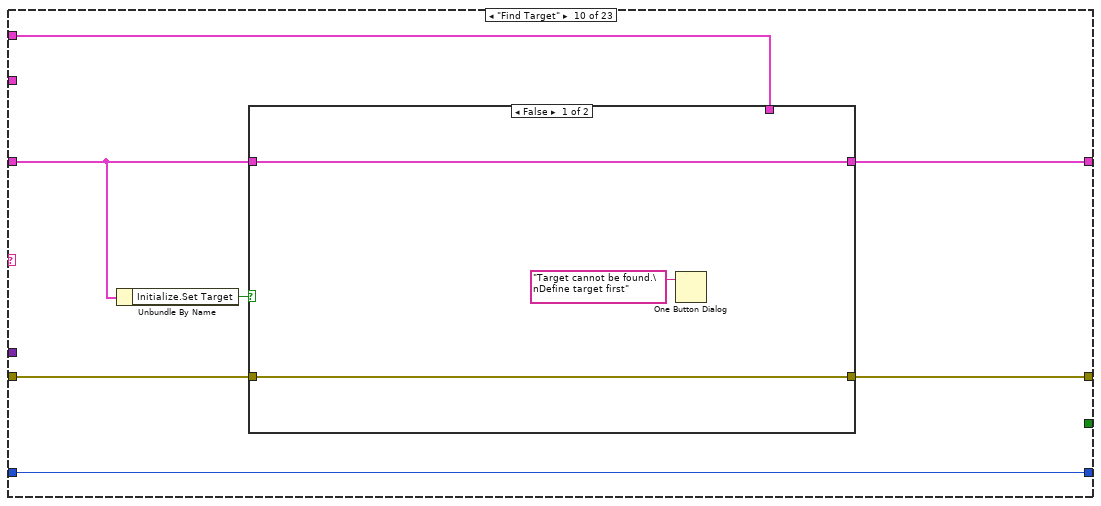
[diagram p15: hidden frame]
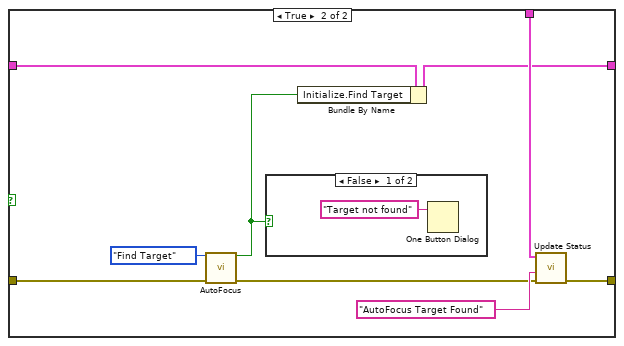
[diagram p16: hidden frame]
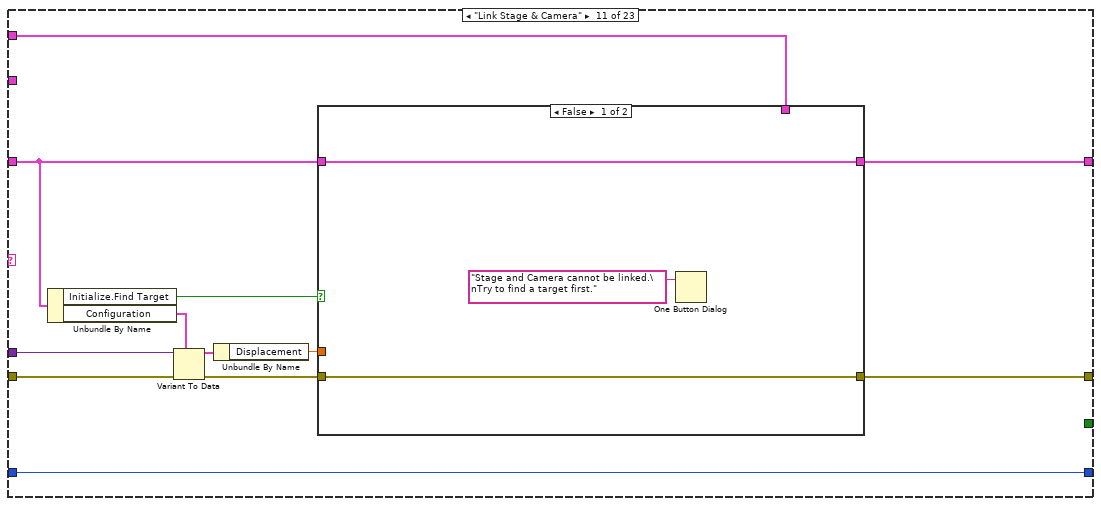
[diagram p18: hidden frame]
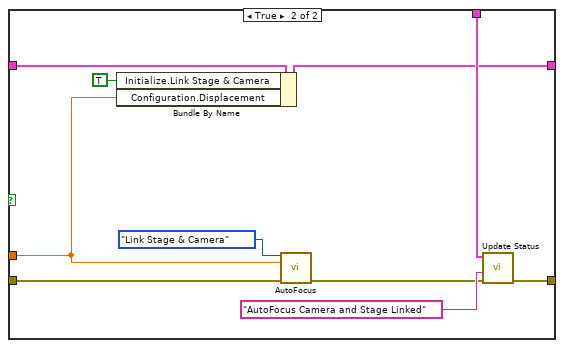
[diagram p19: hidden frame]
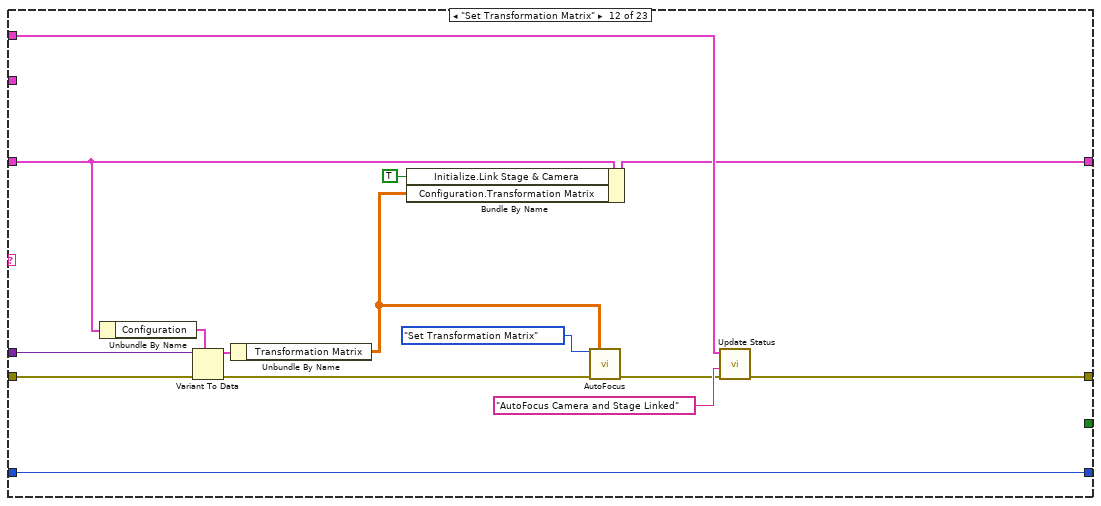
[diagram p20: hidden frame]
diagram:
  w1 = -1  # No Timout
  # "LICENSED MATERIALS – PROPERTY OF IBM\nCopyright IBM Corp. 2016,\nALL RIGHTS RESERVED"
  n1 = call "AutoFocus Data.vi"() -> ("AutoFocus Data"=w2:T58)
  n2 = while "Queued Message Handler for AutoFocus" {
    tunnel: "error in" -> [w24]
    tunnel: [w16] -> w3
    tunnel: "Message Queues out" -> [w20]
    tunnel: "Notifiers" -> [w19]
    tunnel: "IBM OptoElectroMechanics Configuration" -> [w14]
    shift-right: [w11] -> _
    shift-left: w2 -> [w12]
    shift-right: [w8] -> _
    shift-left: w1 -> [w9]
    stop <- w18 stop-if-true
    # "Configurations"
    # "Notifiers"
    # "Message Queues"
    n3 = Unbundle By Name(w20) -> ("AutoFocus"=w15:refnum<queue>)
    n4 = Unbundle By Name(w14) -> ("AutoFocus"=w13:T28)
    n5 = call "Dequeue Message With Timeout.vi"("error in (no error)"=w24, "Timeout in ms (-1)"=w9, "Queue In"=w15) -> ("error out"=w23:errorcluster, "Message Data"=w21:variant, "Message"=w22:string, "timed out?"=w10:bool)  [unwired: 4 in, 1 out]
    n6 = case shown="False" w10 {
      tunnel: w23 -> [w36 w461]
      tunnel: w22 -> [w35 _]
      tunnel: w21 -> [w34 _]
      tunnel: w20 -> [w33 _]
      tunnel: w19 -> [w32 _]
      tunnel: [w31 _] -> w18
      tunnel: [w30 w460] -> w17
      tunnel: w13 -> [w29 _]
      tunnel: w12 -> [w28 w456]
      tunnel: [w27 w456] -> w11
      tunnel: w9 -> [w26 w462]
      tunnel: [w25 w462] -> w8
      frame False {
        n7 = case "Queued Message" shown="\"Focus\"" w35 {
          selector: w35 -> [w40 _ _ _ _ _ _ _ _ _ _ _ _ _ _ _ _ _ _ _ _ _ _]
          tunnel: w36 -> [_ w53 w61 w74 w92 w121 w124 w140 w153 w184 w209 w237 w244 w283 w317 w337 w381 w397 w405 w413 w428 w442 w454]
          tunnel: [w39 w46 w62 w83 w90 w120 w132 w147 w150 w187 w212 w240 w253 w286 w322 w342 w372 w402 w410 w418 w423 w436 w453] -> w30
          tunnel: w34 -> [_ _ _ _ _ w122 _ w134 _ _ w206 w234 w245 w279 _ _ _ _ _ _ w421 _ _]
          tunnel: w33 -> [_ w57 w63 w86 w91 w109 w131 w146 w149 w186 w211 w239 w252 w285 w321 w341 w383 w401 w409 w417 w429 w447 _]
          tunnel: w32 -> [_ _ _ _ w89 w110 _ _ _ _ _ _ w241 _ _ w333 w374 _ _ _ _ w439 w452]
          tunnel: [_ _ _ _ _ _ _ _ _ _ _ _ _ _ _ _ _ _ _ _ _ TRUE ("Priority Message? (F)") _] -> w31
          tunnel: w29 -> [_ w45 _ _ _ _ _ _ _ _ _ _ _ _ _ _ _ _ _ _ _ _ _]
          tunnel: w28 -> [w38 w56 w60 w81 w95 w117 w128 w139 w152 w182 w202 w236 w246 w281 w318 w338 w382 w396 w404 w412 w420 w440 w449]
          tunnel: [w38 w54 w60 w81 w95 w118 w129 w144 w154 w185 w210 w238 w251 w284 w320 w340 w382 w396 w404 w412 w420 w440 w449] -> w27
          tunnel: w26 -> [w37 w44 w58 w75 w88 w108 w123 w133 w148 w181 w201 w226 w250 w275 w314 _ _ w395 w403 w411 w419 w437 w450]
          tunnel: [w37 w44 w58 w75 w88 w108 w123 w133 w148 w181 w201 w226 w250 w275 w314 w334 w380 w395 w403 w411 w419 w437 w450] -> w25
          frame Default {
            # "The Defualt Case run if there is a message that isn't defined in any of the other cases.\nOutput a program error"
            n8 = Format Into String(format string="The invalid message string \"%s\" was  received in the AutoFocus Loop", w40) -> (resulting string=w42:string)  [unwired: 2 in, 1 out]
            n9 = call <vilib>:"Error Cluster From Error Code.vi"("error message (\"\")"=w42, "error code (0)"=5001) -> ("error out"=w39:errorcluster)  [unwired: 2 in, 5 out]
          }
          frame "Initialize" {
            n10 = Unbundle By Name(w57) -> ("AutoFocus"=w51:refnum<queue>, "Message Handler Loop"=w48:refnum<queue>)
            n11 = call "Enqueue Message (Single).vi"("error in (no error)"=w53, "Message"="AutoFocus - Update Refnums", "Message Queue"=w48) -> ("error out"=w50:errorcluster)  [unwired: 1 in, 7 out]
            n12 = call "Enqueue Message (Single).vi"("error in (no error)"=w50, "Message Data"=w45, "Message"="AutoFocus - Set UI", "Message Queue"=w48) -> ("error out"=w47:errorcluster)  [unwired: 7 out]
            n13 = call "Enqueue Message (Single).vi"("error in (no error)"=w47, "Message"="Check if Refnum Update", "Message Queue"=w51) -> ("error out"=w46:errorcluster)  [unwired: 1 in, 7 out]
            n14 = Bundle By Name(cluster=w56, "Configuration"=w45) -> (w54:T58)
          }
          frame "Check if Refnum Update" {
            n15 = Unbundle By Name(w60) -> ("Initialize.Update Refnums"=w59:bool)
            n16 = case shown="False" w59 {
              tunnel: w63 -> [w68 w73]
              tunnel: [w65 w70] -> w62
              tunnel: w61 -> [w64 w69]
              frame True {
                n17 = Unbundle By Name(w68) -> ("AutoFocus"=w66:refnum<queue>)
                n18 = call "Enqueue Message (Single).vi"("error in (no error)"=w64, "Message"="Continue Initialize", "Message Queue"=w66) -> ("error out"=w65:errorcluster)  [unwired: 1 in, 7 out]
              }
              frame False {
                n19 = Unbundle By Name(w73) -> ("AutoFocus"=w71:refnum<queue>)
                n20 = call "Enqueue Message (Single).vi"("error in (no error)"=w69, "Message"="Check if Refnum Update", "Message Queue"=w71) -> ("error out"=w70:errorcluster)  [unwired: 1 in, 7 out]
              }
            }
          }
          frame "Continue Initialize" {
            n21 = Unbundle By Name(w86) -> ("AutoFocus"=w80:refnum<queue>)
            n22 = call "Enqueue Message (Single).vi"("error in (no error)"=w74, "Message"="Allocate Image Memory", "Message Queue"=w80) -> ("error out"=w87:errorcluster)  [unwired: 1 in, 7 out]
            n23 = Unbundle By Name(w81) -> ("Configuration"=w77:T28)
            n24 = call "Enqueue Message (Single).vi"("error in (no error)"=w87, "Message Data"=w77, "Message"="Set Match Criteria", "Message Queue"=w80) -> ("error out"=w79:errorcluster)  [unwired: 7 out]
            n25 = call "Enqueue Message (Single).vi"("error in (no error)"=w79, "Message Data"=w77, "Message"="Set Transformation Matrix", "Message Queue"=w80) -> ("error out"=w78:errorcluster)  [unwired: 7 out]
            n26 = call "Enqueue Message (Single).vi"("error in (no error)"=w78, "Message"="Ready", "Message Queue"=w80) -> ("error out"=w83:errorcluster)  [unwired: 1 in, 7 out]
          }
          frame "Ready" {
            n27 = Unbundle By Name(w95) -> ("Initialize.Allocate Image Memory"=w96:bool, "Initialize.Set Match Criteria"=w93:bool, "Initialize.Update Refnums"=w94:bool)
            n28 = Compound Arithmetic op=AND(w96, w93, w94) -> (w97:bool)
            n29 = case shown="True" w97 {
              tunnel: [w100 w105] -> w90
              tunnel: w92 -> [w99 w104]
              tunnel: w91 -> [w98 _]
              tunnel: w89 -> [_ w103]
              frame False {
                n30 = Unbundle By Name(w98) -> ("AutoFocus"=w102:refnum<queue>)
                n31 = call "Enqueue Message (Single).vi"("error in (no error)"=w99, "Message"="Ready", "Message Queue"=w102) -> ("error out"=w100:errorcluster)  [unwired: 1 in, 7 out]
              }
              frame True {
                n32 = Unbundle By Name(w103) -> ("AutoFocus.Ready"=w106:refnum<notifier>)
                n33 = Send Notification(notification=TRUE, notifier=w106, error in (no error)=w104) -> (error out=w105:errorcluster)  [unwired: 1 out]
              }
            }
          }
          frame "Update Refnums" {
            n34 = Unbundle By Name(w117) -> ("Refnums"=w116:T59)
            n35 = Variant To Data(error in=w121, type=w116, Variant=w122) -> (data=w111:T59, error out=w115:errorcluster)
            n36 = Bundle By Name(cluster=w117, "Initialize.Update Refnums"=TRUE ("Initialization.Update Refnums"), "Refnums"=w111) -> (w118:T58)
            n37 = call "AutoFocus.vi"("Function"=AutoFocus_Functions."Update Refnums", "error in (no error)"=w115, "Refnums"=w111, "Notifiers"=w110, "Message Queues out"=w109) -> ("error out"=w114:errorcluster)  [unwired: 7 in, 3 out]
            n38 = call "Update Status.vi"("error in"=w114, "String"="AutoFocus Refnums updated" ("button name (\"OK\")"), "Message Queues out"=w109) -> ("error out"=w120:errorcluster)  [unwired: 8 out]
          }
          frame "Allocate Image Memory" {
            n39 = Bundle By Name(cluster=w128, "Initialize.Allocate Image Memory"=TRUE ("Initialization.Update Visa Session")) -> (w129:T58)
            n40 = call "AutoFocus.vi"("Function"=AutoFocus_Functions."Allocate Image Memory", "error in (no error)"=w124) -> ("error out"=w125:errorcluster)  [unwired: 10 in, 3 out]
            n41 = call "Update Status.vi"("error in"=w125, "String"="AutoFocus Image Memory Allocated" ("button name (\"OK\")"), "Message Queues out"=w131) -> ("error out"=w132:errorcluster)  [unwired: 8 out]
          }
          frame "Set Match Criteria" {
            n42 = Unbundle By Name(w139) -> ("Configuration"=w137:T28)
            n43 = Variant To Data(error in=w140, type=w137, Variant=w134) -> (data=w136:T28, error out=w138:errorcluster)
            n44 = Unbundle By Name(w136) -> ("Matching Criteria"=w135:T63)
            n45 = Bundle By Name(cluster=w139, "Initialize.Set Match Criteria"=TRUE ("Initialization.Update Visa Session"), "Configuration.Matching Criteria"=w135) -> (w144:T58)
            n46 = call "AutoFocus.vi"("Function"=AutoFocus_Functions."Set Match Criteria", "Matching Criteria"=w135, "error in (no error)"=w138) -> ("error out"=w141:errorcluster)  [unwired: 9 in, 3 out]
            n47 = call "Update Status.vi"("error in"=w141, "String"="AutoFocus Match Criteria Set" ("button name (\"OK\")"), "Message Queues out"=w146) -> ("error out"=w147:errorcluster)  [unwired: 8 out]
          }
          frame "Set Target" {
            n48 = Unbundle By Name(w152) -> ("Initialize.Set Match Criteria"=w151:bool)
            n49 = case shown="True" w151 {
              tunnel: [w157 w168] -> w154
              tunnel: [w156 w165] -> w150
              tunnel: w152 -> [w157 w167]
              tunnel: w153 -> [w156 w163]
              tunnel: w149 -> [_ w166]
              frame False {
                n50 = One Button Dialog(message="Impossible to set target.\nSet matching criteria first") -> ()  [unwired: 1 in, 1 out]
              }
              frame True {
                n51 = call "AutoFocus.vi"("Function"=AutoFocus_Functions."Get ROI", "error in (no error)"=w163) -> ("error out"=w161:errorcluster)  [unwired: 10 in, 3 out]
                n52 = call "DialogTF.vi"("error in (no error)"=w161, "T button name (\"OK\")"="Learn!" ("button name (\"OK\")"), "message"="Ready to setup a Target?\nThis might take a while.\nThank you for your patience.") -> ("error out"=w160:errorcluster, "T button?"=w158:bool)  [unwired: 7 in]
                n53 = case shown="True" w158 {
                  tunnel: [w170 w180] -> w168
                  tunnel: w167 -> [w170 w177]
                  tunnel: w166 -> [_ w175]
                  tunnel: [w169 w174] -> w165
                  tunnel: w160 -> [w169 w173]
                  frame False {
                  }
                  frame True {
                    n54 = call "AutoFocus.vi"("Function"=AutoFocus_Functions."Set Target", "error in (no error)"=w173) -> ("Target Found?"=w172:bool, "error out"=w171:errorcluster)  [unwired: 10 in, 2 out]
                    n55 = Bundle By Name(cluster=w177, "Initialize.Set Target"=TRUE ("Initialization.Update Visa Session"), "Initialize.Find Target"=w172) -> (w180:T58)
                    n56 = call "Update Status.vi"("error in"=w171, "String"="AutoFocus Target Set" ("button name (\"OK\")"), "Message Queues out"=w175) -> ("error out"=w174:errorcluster)  [unwired: 8 out]
                  }
                }
              }
            }
          }
          frame "Find Target" {
            n57 = Unbundle By Name(w182) -> ("Initialize.Set Target"=w183:bool)
            n58 = case shown="False" w183 {
              tunnel: [w188 w199] -> w187
              tunnel: w186 -> [_ w198]
              tunnel: [w189 w191] -> w185
              tunnel: w182 -> [w189 w192]
              tunnel: w184 -> [w188 w194]
              frame False {
                n59 = One Button Dialog(message="Target cannot be found.\nDefine target first") -> ()  [unwired: 1 in, 1 out]
              }
              frame True {
                n60 = call "AutoFocus.vi"("Function"=AutoFocus_Functions."Find Target", "error in (no error)"=w194) -> ("Target Found?"=w193:bool, "error out"=w195:errorcluster)  [unwired: 10 in, 2 out]
                n61 = case shown="False" w193 {
                  frame False {
                    n62 = One Button Dialog(message="Target not found") -> ()  [unwired: 1 in, 1 out]
                  }
                  frame True {
                  }
                }
                n63 = Bundle By Name(cluster=w192, "Initialize.Find Target"=w193) -> (w191:T58)
                n64 = call "Update Status.vi"("error in"=w195, "String"="AutoFocus Target Found" ("button name (\"OK\")"), "Message Queues out"=w198) -> ("error out"=w199:errorcluster)  [unwired: 8 out]
              }
            }
          }
          frame "Link Stage & Camera" {
            n65 = Unbundle By Name(w202) -> ("Initialize.Find Target"=w208:bool, "Configuration"=w205:T28)
            n66 = Variant To Data(error in=w209, type=w205, Variant=w206) -> (data=w204:T28, error out=w207:errorcluster)
            n67 = Unbundle By Name(w204) -> ("Displacement"=w203:dbl)
            n68 = case shown="False" w208 {
              tunnel: [w213 w225] -> w212
              tunnel: w211 -> [_ w224]
              tunnel: [w214 w218] -> w210
              tunnel: w202 -> [w214 w220]
              tunnel: w207 -> [w213 w219]
              tunnel: w203 -> [_ w217]
              frame False {
                n69 = One Button Dialog(message="Stage and Camera cannot be linked.\nTry to find a target first.") -> ()  [unwired: 1 in, 1 out]
              }
              frame True {
                n70 = Bundle By Name(cluster=w220, "Initialize.Link Stage & Camera"=TRUE, "Configuration.Displacement"=w217) -> (w218:T58)
                n71 = call "AutoFocus.vi"("Function"=AutoFocus_Functions."Link Stage & Camera", "Displacement"=w217, "error in (no error)"=w219) -> ("error out"=w221:errorcluster)  [unwired: 9 in, 3 out]
                n72 = call "Update Status.vi"("error in"=w221, "String"="AutoFocus Camera and Stage Linked" ("button name (\"OK\")"), "Message Queues out"=w224) -> ("error out"=w225:errorcluster)  [unwired: 8 out]
              }
            }
          }
          frame "Set Transformation Matrix" {
            n73 = Unbundle By Name(w236) -> ("Configuration"=w233:T28)
            n74 = Variant To Data(error in=w237, type=w233, Variant=w234) -> (data=w232:T28, error out=w235:errorcluster)
            n75 = Unbundle By Name(w232) -> ("Transformation Matrix"=w228:T30)
            n76 = Bundle By Name(cluster=w236, "Initialize.Link Stage & Camera"=TRUE, "Configuration.Transformation Matrix"=w228) -> (w238:T58)
            n77 = call "AutoFocus.vi"("Function"=AutoFocus_Functions."Set Transformation Matrix", "Set Inverse Matrix"=w228, "error in (no error)"=w235) -> ("error out"=w229:errorcluster)  [unwired: 9 in, 3 out]
            n78 = call "Update Status.vi"("error in"=w229, "String"="AutoFocus Camera and Stage Linked" ("button name (\"OK\")"), "Message Queues out"=w239) -> ("error out"=w240:errorcluster)  [unwired: 8 out]
          }
          frame "Focus" {
            n79 = Unbundle By Name(w246) -> ("Initialize.Find Target"=w247:bool, "Configuration"=w249:T28)
            n80 = Variant To Data(error in=w244, type=w249, Variant=w245) -> (data=w248:T28, error out=w243:errorcluster)
            n81 = Unbundle By Name(w248) -> ("Z Scan Parameters"=w242:T29)
            n82 = case shown="True" w247 {
              tunnel: [w254 w268] -> w253
              tunnel: w252 -> [_ w267]
              tunnel: [w255 w262] -> w251
              tunnel: w246 -> [w255 w263]
              tunnel: w243 -> [w254 w264]
              tunnel: w242 -> [_ w258]
              tunnel: w241 -> [_ w257]
              frame False {
                n83 = One Button Dialog(message="Stage and Camera cannot be linked.\nTry to find a target first.") -> ()  [unwired: 1 in, 1 out]
              }
              frame True {
                n84 = call "AutoFocus.vi"("Function"=AutoFocus_Functions."Focus (Turning Points)", "Z Scan Parameters"=w258, "error in (no error)"=w264) -> ("Target Found?"=w259:bool, "error out"=w260:errorcluster)  [unwired: 9 in, 2 out]
                n85 = case shown="True" w259 {
                  tunnel: ["Autofocus did not find the Target" ("button name (\"OK\")") "AutoFocus Image in Focus" ("button name (\"OK\")")] -> w266
                  tunnel: [w270 w274] -> w261
                  tunnel: w260 -> [w270 w271]
                  tunnel: w257 -> [_ w273]
                  frame False {
                  }
                  frame True {
                    n86 = call "ComplexAlign.vi"("error in (no error)"=w271, "Notifiers"=w273) -> ("error out"=w274:errorcluster)  [unwired: 9 in]
                  }
                }
                n87 = Bundle By Name(cluster=w263, "Configuration.Z Scan Parameters"=w258) -> (w262:T58)
                n88 = call "Update Status.vi"("error in"=w261, "String"=w266, "Message Queues out"=w267) -> ("error out"=w268:errorcluster)  [unwired: 8 out]
              }
            }
          }
          frame "Find Focus" {
            n89 = Unbundle By Name(w281) -> ("Initialize.Find Target"=w282:bool, "Configuration"=w278:T28)
            n90 = Variant To Data(error in=w283, type=w278, Variant=w279) -> (data=w277:T28, error out=w280:errorcluster)
            n91 = Unbundle By Name(w277) -> ("Z Scan Parameters"=w276:T29)
            n92 = case shown="True" w282 {
              tunnel: [w287 w296] -> w286
              tunnel: w285 -> [_ w295]
              tunnel: [w288 w304] -> w284
              tunnel: w281 -> [w288 w305]
              tunnel: w280 -> [w287 w299]
              tunnel: w276 -> [_ w303]
              frame False {
                n93 = One Button Dialog(message="Stage and Camera cannot be linked.\nTry to find a target first.") -> ()  [unwired: 1 in, 1 out]
              }
              frame True {
                n94 = Bundle By Name(cluster=w305, "Configuration.Z Scan Parameters"=w303) -> (w304:T58)
                n95 = call "AutoFocus.vi"("Function"=AutoFocus_Functions."Find Focus", "Z Scan Parameters"=w303, "error in (no error)"=w299) -> ("error out"=w302:errorcluster)  [unwired: 9 in, 3 out]
                n96 = call "AutoFocus.vi"("Function"=AutoFocus_Functions."Grab Image", "error in (no error)"=w302) -> ("error out"=w298:errorcluster)  [unwired: 10 in, 3 out]
                n97 = call "AutoFocus.vi"("Function"=AutoFocus_Functions."Set ROI", "error in (no error)"=w298) -> ("error out"=w292:errorcluster)  [unwired: 10 in, 3 out]
                n98 = call "DialogTF.vi"("error in (no error)"=w292, "message"="Do you want to redefine the target?\nThis might take a while.\nThank you for your patience.") -> ("error out"=w291:errorcluster, "T button?"=w290:bool)  [unwired: 8 in]
                n99 = case shown="True" w290 {
                  tunnel: AutoFocus_Functions."Set Target" ("Function") -> [_ w313]
                  tunnel: [w307 w310] -> w296
                  tunnel: w291 -> [w307 w312]
                  tunnel: w295 -> [_ w309]
                  tunnel: "AutoFocus Target Optimized" ("button name (\"OK\")") -> [_ w308]
                  frame False {
                  }
                  frame True {
                    n100 = call "AutoFocus.vi"("Function"=w313, "error in (no error)"=w312) -> ("error out"=w311:errorcluster)  [unwired: 10 in, 3 out]
                    n101 = call "Update Status.vi"("error in"=w311, "String"=w308, "Message Queues out"=w309) -> ("error out"=w310:errorcluster)  [unwired: 8 out]
                  }
                }
              }
            }
          }
          frame "Align" {
            n102 = Unbundle By Name(w318) -> ("Initialize.Find Target"=w315:bool, "Initialize.Link Stage & Camera"=w319:bool)
            n103 = Compound Arithmetic op=AND(w315, w319) -> (w316:bool)
            n104 = case shown="True" w316 {
              tunnel: [w323 w332] -> w322
              tunnel: w321 -> [_ w331]
              tunnel: [w324 w326] -> w320
              tunnel: w318 -> [w324 w326]
              tunnel: w317 -> [w323 w327]
              frame False {
                n105 = One Button Dialog(message="Cannot compensate misallignment.\nSet Target first , or link stage and camera.") -> ()  [unwired: 1 in, 1 out]
              }
              frame True {
                n106 = call "AutoFocus.vi"("Function"=AutoFocus_Functions."Align", "error in (no error)"=w327) -> ("error out"=w328:errorcluster)  [unwired: 10 in, 3 out]
                n107 = call "Update Status.vi"("error in"=w328, "String"="AutoFocus compensated the sample misalignment" ("button name (\"OK\")"), "Message Queues out"=w331) -> ("error out"=w332:errorcluster)  [unwired: 8 out]
              }
            }
          }
          frame "Start Tracking" {
            n108 = Unbundle By Name(w338) -> ("Initialize.Find Target"=w335:bool, "Initialize.Link Stage & Camera"=w339:bool)
            n109 = Compound Arithmetic op=AND(w335, w339) -> (w336:bool)
            n110 = case shown="True" w336 {
              tunnel: [w344 w349] -> w342
              tunnel: w341 -> [_ w359]
              tunnel: [w345 w355] -> w340
              tunnel: w338 -> [w345 w355]
              tunnel: w337 -> [w344 w356]
              tunnel: [w343 w357] -> w334
              tunnel: w333 -> [_ w347]
              frame False {
                w343 = -1  # No Timout
                n111 = One Button Dialog(message="Cannot Track device.\nSet Target first , or link stage and camera.") -> ()  [unwired: 1 in, 1 out]
              }
              frame True {
                w357 = 500  # Timout
                n112 = Unbundle By Name(w355) -> ("Refnums.Tracking"=w354:refnum<vi>)
                n113 = Not A Number/Path/Refnum?(number/path/refnum=w354) -> (NaN/Path/Refnum?=w353:bool)
                n114 = case shown="False" w353 {
                  tunnel: w356 -> [w369 w370]
                  tunnel: [w368 w370] -> w350
                  tunnel: w354 -> [w367 _]
                  frame False {
                    n115 = property class="Bool (strict)"(reference=w367, error in=w369, "Value"=TRUE) -> (error out=w368:errorcluster)  [unwired: 1 out]
                  }
                  frame True {
                  }
                }
                n116 = Unbundle By Name(w347) -> ("AutoFocus.Status"=w351:refnum<notifier>)
                n117 = Not A Number/Path/Refnum?(number/path/refnum=w351) -> (NaN/Path/Refnum?=w352:bool)
                n118 = case shown="False" w352 {
                  tunnel: w350 -> [w364 w365]
                  tunnel: [w363 w365] -> w348
                  tunnel: w351 -> [w362 _]
                  frame False {
                    n119 = Send Notification(notification="Tracking Started", notifier=w362, error in (no error)=w364) -> (error out=w363:errorcluster)  [unwired: 1 out]
                  }
                  frame True {
                  }
                }
                n120 = call "Update Status.vi"("error in"=w350, "String"="AutoFocus Tracking Started" ("button name (\"OK\")"), "Message Queues out"=w359) -> ("error out"=w360:errorcluster)  [unwired: 8 out]
                n121 = Merge Errors(w348, w360) -> (w349:errorcluster)
              }
            }
          }
          frame "Stop Tracking" {
            w380 = -1  # Timout
            n122 = Unbundle By Name(w382) -> ("Refnums.Tracking"=w378:refnum<vi>)
            n123 = Not A Number/Path/Refnum?(number/path/refnum=w378) -> (NaN/Path/Refnum?=w377:bool)
            n124 = case shown="False" w377 {
              tunnel: w381 -> [w393 w394]
              tunnel: [w392 w394] -> w373
              tunnel: w378 -> [w391 _]
              frame False {
                n125 = property class="Bool (strict)"(reference=w391, error in=w393, "Value"=FALSE) -> (error out=w392:errorcluster)  [unwired: 1 out]
              }
              frame True {
              }
            }
            n126 = Unbundle By Name(w374) -> ("AutoFocus.Status"=w375:refnum<notifier>)
            n127 = Not A Number/Path/Refnum?(number/path/refnum=w375) -> (NaN/Path/Refnum?=w376:bool)
            n128 = case shown="False" w376 {
              tunnel: w373 -> [w388 w389]
              tunnel: [w387 w389] -> w371
              tunnel: w375 -> [w386 _]
              frame False {
                n129 = Send Notification(notification="Tracking Stopped", notifier=w386, error in (no error)=w388) -> (error out=w387:errorcluster)  [unwired: 1 out]
              }
              frame True {
              }
            }
            n130 = call "Update Status.vi"("error in"=w373, "String"="AutoFocus Tracking Stopped" ("button name (\"OK\")"), "Message Queues out"=w383) -> ("error out"=w384:errorcluster)  [unwired: 8 out]
            n131 = Merge Errors(w371, w384) -> (w372:errorcluster)
          }
          frame "Grab Image" {
            n132 = call "AutoFocus.vi"("Function"=AutoFocus_Functions."Grab Image", "error in (no error)"=w397) -> ("error out"=w398:errorcluster)  [unwired: 10 in, 3 out]
            n133 = call "Update Status.vi"("error in"=w398, "String"="AutoFocus Image Acquired" ("button name (\"OK\")"), "Message Queues out"=w401) -> ("error out"=w402:errorcluster)  [unwired: 8 out]
          }
          frame "Get ROI" {
            n134 = call "AutoFocus.vi"("Function"=AutoFocus_Functions."Get ROI", "error in (no error)"=w405) -> ("error out"=w406:errorcluster)  [unwired: 10 in, 3 out]
            n135 = call "Update Status.vi"("error in"=w406, "String"="AutoFocus Region of Interest Updated" ("button name (\"OK\")"), "Message Queues out"=w409) -> ("error out"=w410:errorcluster)  [unwired: 8 out]
          }
          frame "Set ROI" {
            n136 = call "AutoFocus.vi"("Function"=AutoFocus_Functions."Set ROI", "error in (no error)"=w413) -> ("error out"=w414:errorcluster)  [unwired: 10 in, 3 out]
            n137 = call "Update Status.vi"("error in"=w414, "String"="AutoFocus Region of Interest Set" ("button name (\"OK\")"), "Message Queues out"=w417) -> ("error out"=w418:errorcluster)  [unwired: 8 out]
          }
          frame "Error" {
            # "Clear Errors to avoid getting stuck \nin repeating this case"
            # "Add here Cases that are handled \nalready by the Message Handler Loop"
            n138 = Variant To Data(error in=w428, type=errorcluster {"status"=FALSE, "code"=0, "source"=""} ("error out"), Variant=w421) -> (data=w427:errorcluster, error out=w426:errorcluster)
            n139 = Merge Errors(w427, w426) -> (w425:errorcluster)
            n140 = Unbundle By Name(w429) -> ("Message Handler Loop"=w431:refnum<queue>)
            n141 = Unbundle By Name(w425) -> ("code"=w422:i32)
            n142 = case shown="Default" w422 {
              tunnel: w431 -> [w435]
              tunnel: w425 -> [w433]
              tunnel: [w432] -> w424
              frame Default {
                n143 = call "Enqueue Message (Single).vi"("Message Data"=w433, "Message"="Error", "Message Queue"=w435) -> ("error out"=w432:errorcluster)  [unwired: 1 in, 7 out]
              }
            }
            n144 = call <vilib>:"Clear Errors.vi"("error in (no error)"=w424) -> ("error out"=w423:errorcluster)  [unwired: 1 in, 5 out]
          }
          frame "Exit" {
            # "Stop the VI"
            n145 = call "AutoFocus.vi"("Function"=AutoFocus_Functions."Free Image Memory", "error in (no error)"=w442) -> ("error out"=w441:errorcluster)  [unwired: 10 in, 3 out]
            n146 = Unbundle By Name(w447) -> ("AutoFocus"=w448:refnum<queue>)
            n147 = Release Queue(queue=w448, error in (no error)=w441) -> (error out=w446:errorcluster)  [unwired: 3 out]
            n148 = Unbundle By Name(w439) -> ("AutoFocus.Exit"=w445:refnum<notifier>)
            n149 = Send Notification(notification=FALSE ("Priority Message? (F)"), notifier=w445, error in (no error)=w446) -> (error out=w436:errorcluster)  [unwired: 1 out]
          }
          frame "Notify Status" {
            n150 = Unbundle By Name(w452) -> ("AutoFocus.Instrument Data"=w451:refnum<notifier>)
            n151 = Send Notification(notification=w449, notifier=w451, error in (no error)=w454) -> (error out=w453:errorcluster)  [unwired: 1 out]
          }
        }
      }
      frame True {
        # "Tracking device"
        n152 = Unbundle By Name(w456) -> ("Initialize.Find Target"=w458:bool, "Initialize.Link Stage & Camera"=w459:bool, "Initialize.Set Target"=w457:bool)
        n153 = Compound Arithmetic op=AND(w458, w459, w457) -> (w455:bool)
        n154 = case shown="True" w455 {
          tunnel: w461 -> [w463 w465]
          tunnel: [w463 w464] -> w460
          frame False {
          }
          frame True {
            n155 = call "AutoFocus.vi"("Function"=AutoFocus_Functions."Align", "error in (no error)"=w465) -> ("error out"=w464:errorcluster)  [unwired: 10 in, 3 out]
          }
        }
      }
    }
    n156 = call "Message Handling Loop.vi"("error in (no error)"=w17, "Message Queue"=w15) -> ("dup error in"=w16:errorcluster)  [unwired: 9 out]
  }
  "error out" <- w3
